vi "运维调试_总磷总氮.vi"() -> ()   [LabVIEW 2016, in "斯坦道总磷.lvlib"]
uses:
  <vilib>/Utility/miscctls.llb/LVStringsAndValuesArrayTypeDef_U16.ctl
  <vilib>/Utility/miscctls.llb/LVPointTypeDef.ctl
  <vilib>/Plasmionique/MB Master/MB_Master/MB_Master.lvclass
  <vilib>/Utility/config.llb/NI_LVConfig.lvlib
  <vilib>/ptbypt/NI_PtbyPt.lvlib
panel:
  in  "灯值调整":bool
  in  "测试量程配置":T1
  in  "启动参数设置":bool
  out "固件版本号":string
  in  "定时设置":cluster{"启动":bool, "控制命令":T2, "测量参数":T3}(xcontrol)
  out "模块版本号":string
  out "温度2":sgl
  out "温度1":sgl
  out "ADC":sgl
  out "F3":sgl format="%#.6f"
  out "F2":sgl format="%#.6f"
  out "F1":sgl format="%#.6f"
  out "F0":sgl format="%#.6f"
  out "运行状态":T4 {"数据时间:" format="%<%y/%m/%d %H:%M:%S>T"; "仪器时间:" format="%<%y/%m/%d %H:%M:%S>T"}
  in  "单选按钮":enum32{"COD", "NH3N", "TN", "TP"}(radio)=enum."TN"
  in  "仪器参数":bool
  out "二级权限":bool
  out "一级权限":bool
  out "输入密码":u32
  out "布尔":bool
  in  "流程固件":bool
  in  "量程参数读取":T5
  in  "模块启用":bool
  in  "串口设置":bool
  in  "公式一键写入":bool
  in  "流程路径":path=path "data/流程.xml"
  in  "曲线模型":cluster{"X^2":dbl, "X":dbl, "B":dbl, "r^2":dbl}(xcontrol)
  out "字符串 2":string
  in  "质控参数设置":bool
  in  "数组":string[](array[string])
  in  "量程切换阈值写入":bool
  in  "量程切换阈值读取":bool
  in  "参数下拉列表":enum16{"COD", "氨氮", "总氮", "总磷"}(ring)
  in  "量程下拉列表":enum16{"低量程", "高量程"}(ring)
  in  "测量模式下拉列表":enum16{"水样测量", "零点核查", "跨度核查", "标样核查", "加标回收"}(ring)
  in  "公式":cluster{"X^2":dbl, "X":dbl, "b":dbl}
  in  "写公式":bool
  in  "读公式":bool
  in  "返回":bool
  in  "参数设置":bool
  out "集成报警信息":string
  in  "停止":bool
  in  "手动启动":bool
  in  "单步测试":bool
  out "多列列表框":i32(listbox)
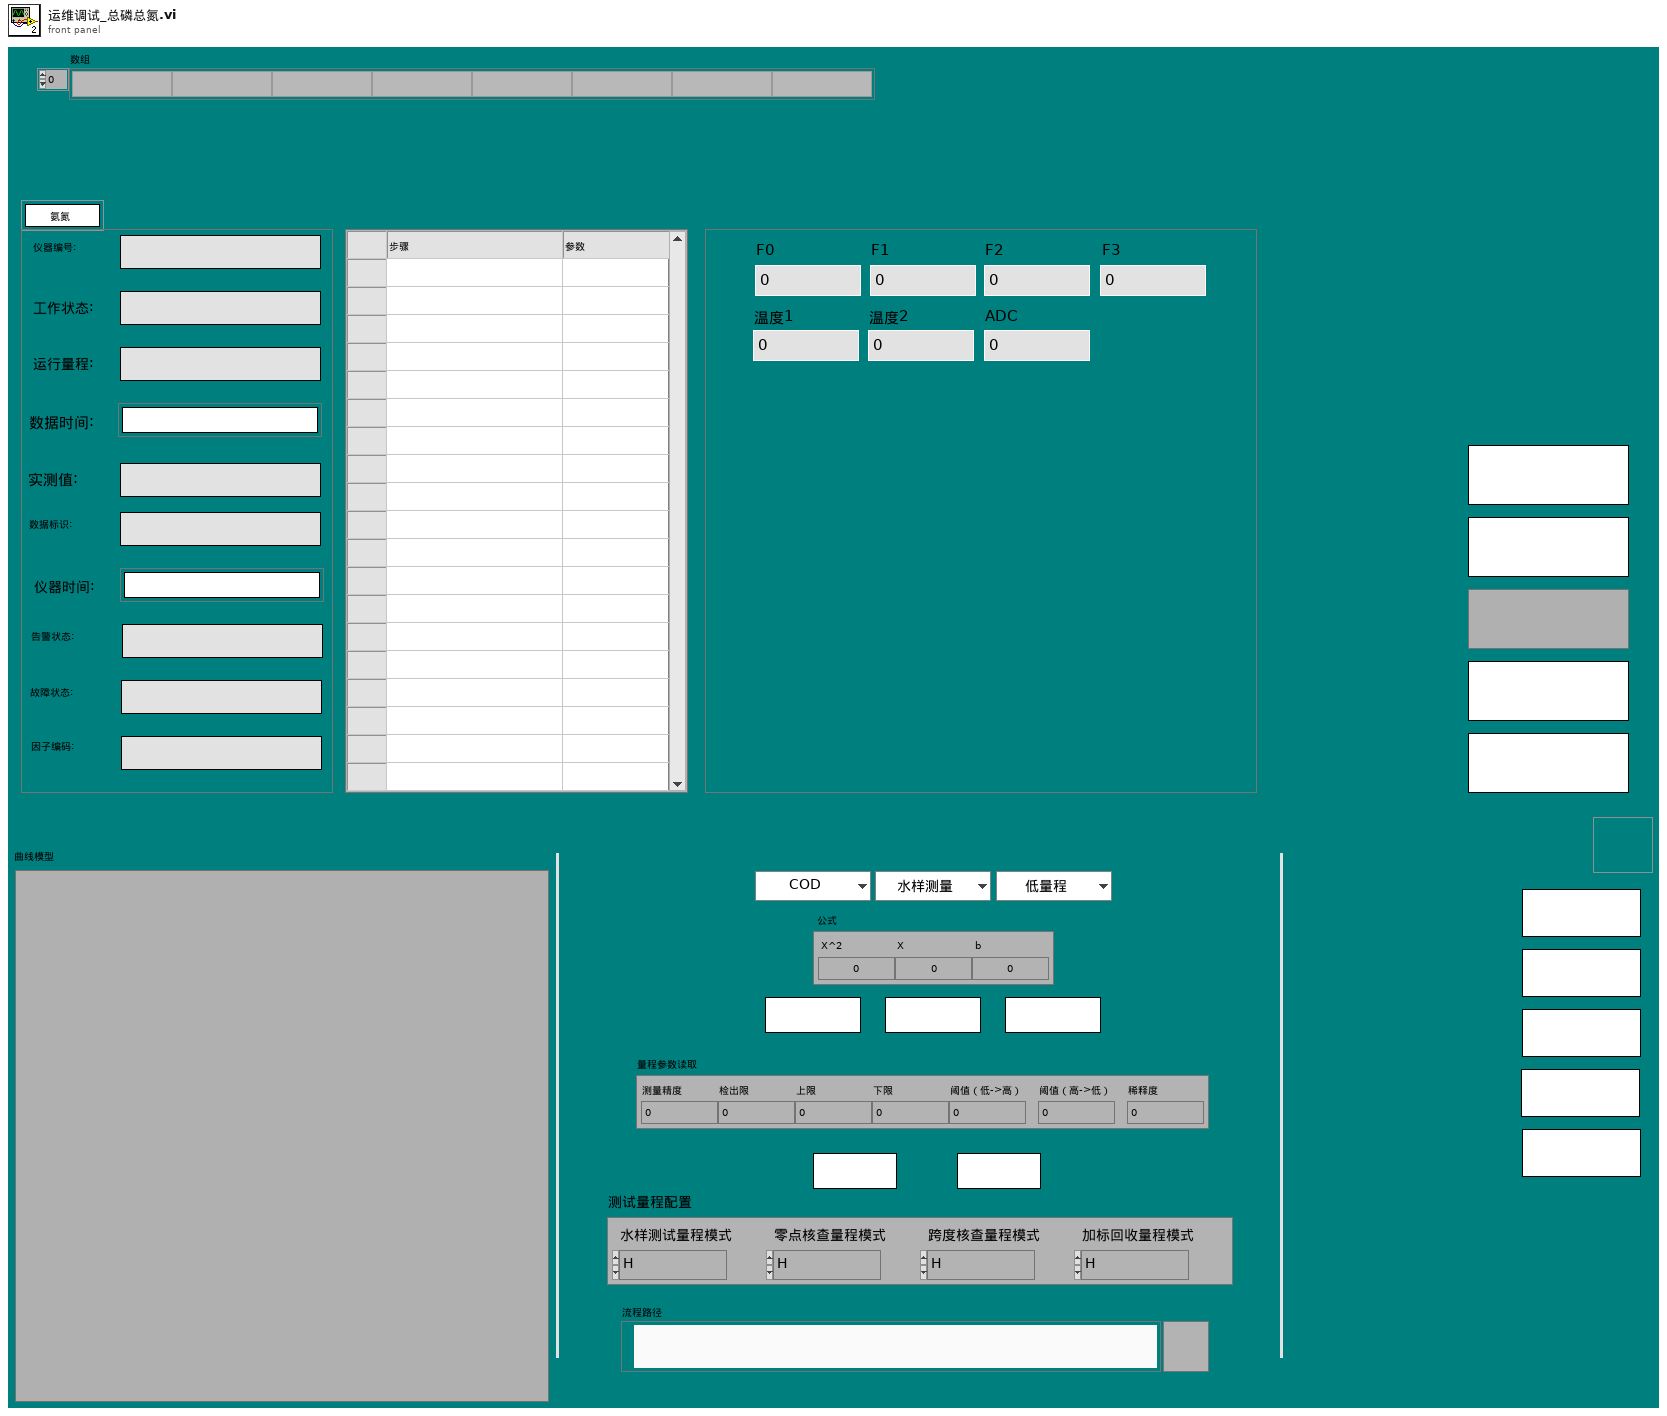
[diagram p1: front panel]
types:
  T1 = cluster{"水样测试量程模式":enum16{"H", "L", "AUTO"}, "空白核查量程模式":enum16{"H", "L", "AUTO"}, "跨度核查量程模式":enum16{"H", "L", "AUTO"}, "跨度核查量程模式 2":enum16{"H", "L", "AUTO"}}
  T2 = typedef "定时设置.xctl/国标控制命令.ctl" = enum16{"启动测量", "标样核查", "零点核查", "跨度核查", "空白测试", "平行样测试", "加标回收", "空白校准", "标样校准", "初始化（清洗）", "停止测试", "仪器重启", "校时", "模式设置", "测量间隔设置"}
  T3 = typedef "定时设置.xctl/测量参数.ctl" = u16
  T4 = cluster{"仪器编号:":string, "工作状态:":string, "运行量程: ":string, "数据时间:":timestamp, "实测值:":string, "数据标识: ":string, "仪器时间:":timestamp, "告警状态: ":string, "故障状态:  ":string, "因子编码:":string}
  T5 = cluster{"测量精度":dbl, "检出限":dbl, "上限":dbl, "下限":dbl, "阈值（低->高）":dbl, "阈值（高->低）":dbl, "稀释度":dbl}
  T6 = cluster{"时间源选择":enum16{"系统时间源", "仪器时间源"}, "外部时间源":timestamp}
  T7 = cluster{"系统时间":timestamp, "工作状态":enum16{"空闲", "水样测试", "标样核查", "零点核查", "跨度核查", "空白测试", "平行样测试", "加标回收", "空白校准", "标样校准", "初始化（清洗）"}, "测量模式":enum16{"待机", "连续模式", "周期模式", "定点模式", "受控模式", "手动模式"}, "告警代码":u16, "故障代码":u16, "日志代码":u16, "软件版本":u16, "F0":sgl, "F1":sgl, "F2":sgl, "F3":sgl, "T":sgl, "H":sgl, "id":u16, "flowid":u16, "量程":u16, "总磷控温温度1":sgl, "营养盐控温温度2":sgl, "ADC":sgl}
  T8 = enum32{"Bad", "Idle", "Run top level", "Running"}
  T9 = enum16{"空闲", "水样测试", "标样核查", "零点核查", "跨度核查", "空白测试", "平行样测试", "加标回收", "空白校准", "标样校准", "初始化（清洗）"}
  T10 = cluster{"水样测试量程模式":enum16{"H", "L", "AUTO"}, "空白核查量程模式":enum16{"H", "L", "AUTO"}, "跨度核查量程模式":enum16{"H", "L", "AUTO"}, "加标回收量程模式":enum16{"H", "L", "AUTO"}}
  T11 = typedef "LVStringsAndValuesArrayTypeDef_U16.ctl" = cluster{"String":string, "Value":u16}[]
  T12 = cluster{"COD":bool, "氨氮":bool, "总氮":bool, "总磷":bool}
  T13 = typedef "LVPointTypeDef.ctl" = cluster{"Horizontal":i16, "Vertical":i16}
  T14 = cluster{"因子编码":u32, "单位":u16, "标样参考值":sgl, "水样数据时间":timestamp, "水样实测值":sgl, "水样数据标识":string, "标样数据时间":timestamp, "标样实测值":sgl, "标样数据标识":string, "空白数据时间":timestamp, "空白实测值":sgl, "空白数据标识":string, "零点核查数据时间":timestamp, "零点核查实测值":sgl, "零点核查数据标识":string, "跨度核查数据时间":timestamp, "跨度核查实测值":sgl, "跨度核查数据标识":string, "加标回收数据时间":timestamp, "加标回收实测值":sgl, "加标回收数据标识":string, "平行样数据时间":timestamp, "平行样实测值":sgl, "平行样数据标识":string, "F0":sgl, "F1":sgl, "F2":sgl, "F3":sgl, "F4":sgl, "F5":sgl, "F6":sgl, "F7":sgl, "温度":sgl, "湿度":sgl, "X值":sgl, "fidrange":u16}
  T15 = cluster{"时间标识":timestamp, "设备":string, "日志信息":string, "备注":string}
  T16 = cluster{"参数":string, "报警内容":string, "报警分析":string}
  T17 = typedef "NI_LVConfig.lvlib/Config Data RefNum.ctl" = refnum<k1>
  T18 = cluster{"启动模式":enum16{"跨度核查", "水样测量", "空白核查", "标样核查", "加标回收"}, "启动参数":u16, "量程":enum16{"低量程", "高量程"}}
  T19 = cluster{"时间标识":timestamp, "设备":string, "日志信息":string, "流程参数":string}
  T20 = typedef "LVRowAndColumnUnsignedTypeDef.ctl" = cluster{"Row":u32, "Column":u32}
  T21 = cluster{"Major":u16, "Minor":u16, "Fix":u16, "Build":u16}
  T22 = cluster{"站号":u16, "量程切换":enum32{"H", "L", "AUTO"}, "控制命令":enum16{"启动测量", "标样核查", "零点核查", "跨度核查", "空白测试", "平行样测试", "加标回收", "空白校准", "标样校准", "初始化（清洗）", "停止测试", "仪器重启", "校时", "模式设置", "测量间隔设置"}, "模式设置":enum16{"待机", "连续模式", "周期模式", "定点模式", "受控模式", "手动模式"}, "测量间隔":u16}
  T23 = cluster{"参数下拉列表":enum16{"COD", "氨氮", "总氮", "总磷"}, "测量模式下拉列表":enum16{"水样测量", "零点核查", "跨度核查", "标样核查", "加标回收"}, "量程下拉列表":enum16{"低量程", "高量程"}}
  T24 = cluster{"被复制模型":cluster{"参数":u8, "测量模式":u8, "量程":u8}, "被覆盖模型":cluster{"参数":u8, "测量模式":u8, "量程":u8}[]}
  T25 = cluster{"总磷跨度值":dbl, "总磷零点标准液浓度":dbl, "总磷跨度标准液浓度":dbl, "总磷标准液标准浓度":dbl, "总氮跨度值":dbl, "总氮零点标准液浓度":dbl, "总氮跨度标准液浓度":dbl, "总氮标准液标准浓度":dbl, "COD跨度值":dbl, "COD零点标准液浓度":dbl, "COD跨度标准液浓度":dbl, "COD标准液标准浓度":dbl, "氨氮跨度值":dbl, "氨氮零点标准液浓度":dbl, "氨氮跨度标准液浓度":dbl, "氨氮标准液标准浓度":dbl}
  T26 = cluster{"测量量程":dbl, "测量精度":dbl, "测量间隔":dbl, "消解温度":dbl, "消解时长":dbl, "空白校准时间":timestamp, "曲线截距":dbl, "曲线斜率":dbl, "测量检出限":dbl, "测量信号值":dbl, "线性相关系数":dbl, "二次多项式系数":dbl, "标样校准时间":timestamp, "稀释倍数":dbl, "三项式系数":dbl, "空白标定系数":dbl, "量程系数":dbl, "F0/ORPA":dbl, "F1/ORPB":dbl, "F2/ORPK":dbl, "F3":dbl, "F4":dbl, "F5":dbl, "F6":dbl, "F7":dbl, "X0/滴定数":dbl, "量程":dbl}
  T27 = cluster{"COD仪器参数":cluster{"测量量程":dbl, "测量精度":dbl, "测量间隔":dbl, "消解温度":dbl, "消解时长":dbl, "空白校准时间":timestamp, "曲线截距":dbl, "曲线斜率":dbl, "测量检出限":dbl, "测量信号值":dbl, "线性相关系数":dbl, "二次多项式系数":dbl, "标样校准时间":timestamp, "稀释倍数":dbl, "三项式系数":dbl, "空白标定系数":dbl, "量程系数":dbl, "F0/ORPA":dbl, "F1/ORPB":dbl, "F2/ORPK":dbl, "F3":dbl, "F4":dbl, "F5":dbl, "F6":dbl, "F7":dbl, "X0/滴定数":dbl, "量程":dbl}, "氨氮仪器参数":cluster{"测量量程":dbl, "测量精度":dbl, "测量间隔":dbl, "消解温度":dbl, "消解时长":dbl, "空白校准时间":timestamp, "曲线截距":dbl, "曲线斜率":dbl, "测量检出限":dbl, "测量信号值":dbl, "线性相关系数":dbl, "二次多项式系数":dbl, "标样校准时间":timestamp, "稀释倍数":dbl, "三项式系数":dbl, "空白标定系数":dbl, "量程系数":dbl, "F0/ORPA":dbl, "F1/ORPB":dbl, "F2/ORPK":dbl, "F3":dbl, "F4":dbl, "F5":dbl, "F6":dbl, "F7":dbl, "X0/滴定数":dbl, "量程":dbl}, "总氮仪器参数":cluster{"测量量程":dbl, "测量精度":dbl, "测量间隔":dbl, "消解温度":dbl, "消解时长":dbl, "空白校准时间":timestamp, "曲线截距":dbl, "曲线斜率":dbl, "测量检出限":dbl, "测量信号值":dbl, "线性相关系数":dbl, "二次多项式系数":dbl, "标样校准时间":timestamp, "稀释倍数":dbl, "三项式系数":dbl, "空白标定系数":dbl, "量程系数":dbl, "F0/ORPA":dbl, "F1/ORPB":dbl, "F2/ORPK":dbl, "F3":dbl, "F4":dbl, "F5":dbl, "F6":dbl, "F7":dbl, "X0/滴定数":dbl, "量程":dbl}, "总磷仪器参数":cluster{"测量量程":dbl, "测量精度":dbl, "测量间隔":dbl, "消解温度":dbl, "消解时长":dbl, "空白校准时间":timestamp, "曲线截距":dbl, "曲线斜率":dbl, "测量检出限":dbl, "测量信号值":dbl, "线性相关系数":dbl, "二次多项式系数":dbl, "标样校准时间":timestamp, "稀释倍数":dbl, "三项式系数":dbl, "空白标定系数":dbl, "量程系数":dbl, "F0/ORPA":dbl, "F1/ORPB":dbl, "F2/ORPK":dbl, "F3":dbl, "F4":dbl, "F5":dbl, "F6":dbl, "F7":dbl, "X0/滴定数":dbl, "量程":dbl}}
  T28 = cluster{"测量精度":u16, "检出限":dbl, "上限":dbl, "下限":dbl, "阈值（低->高）":dbl, "阈值（高->低）":dbl, "稀释度":dbl}
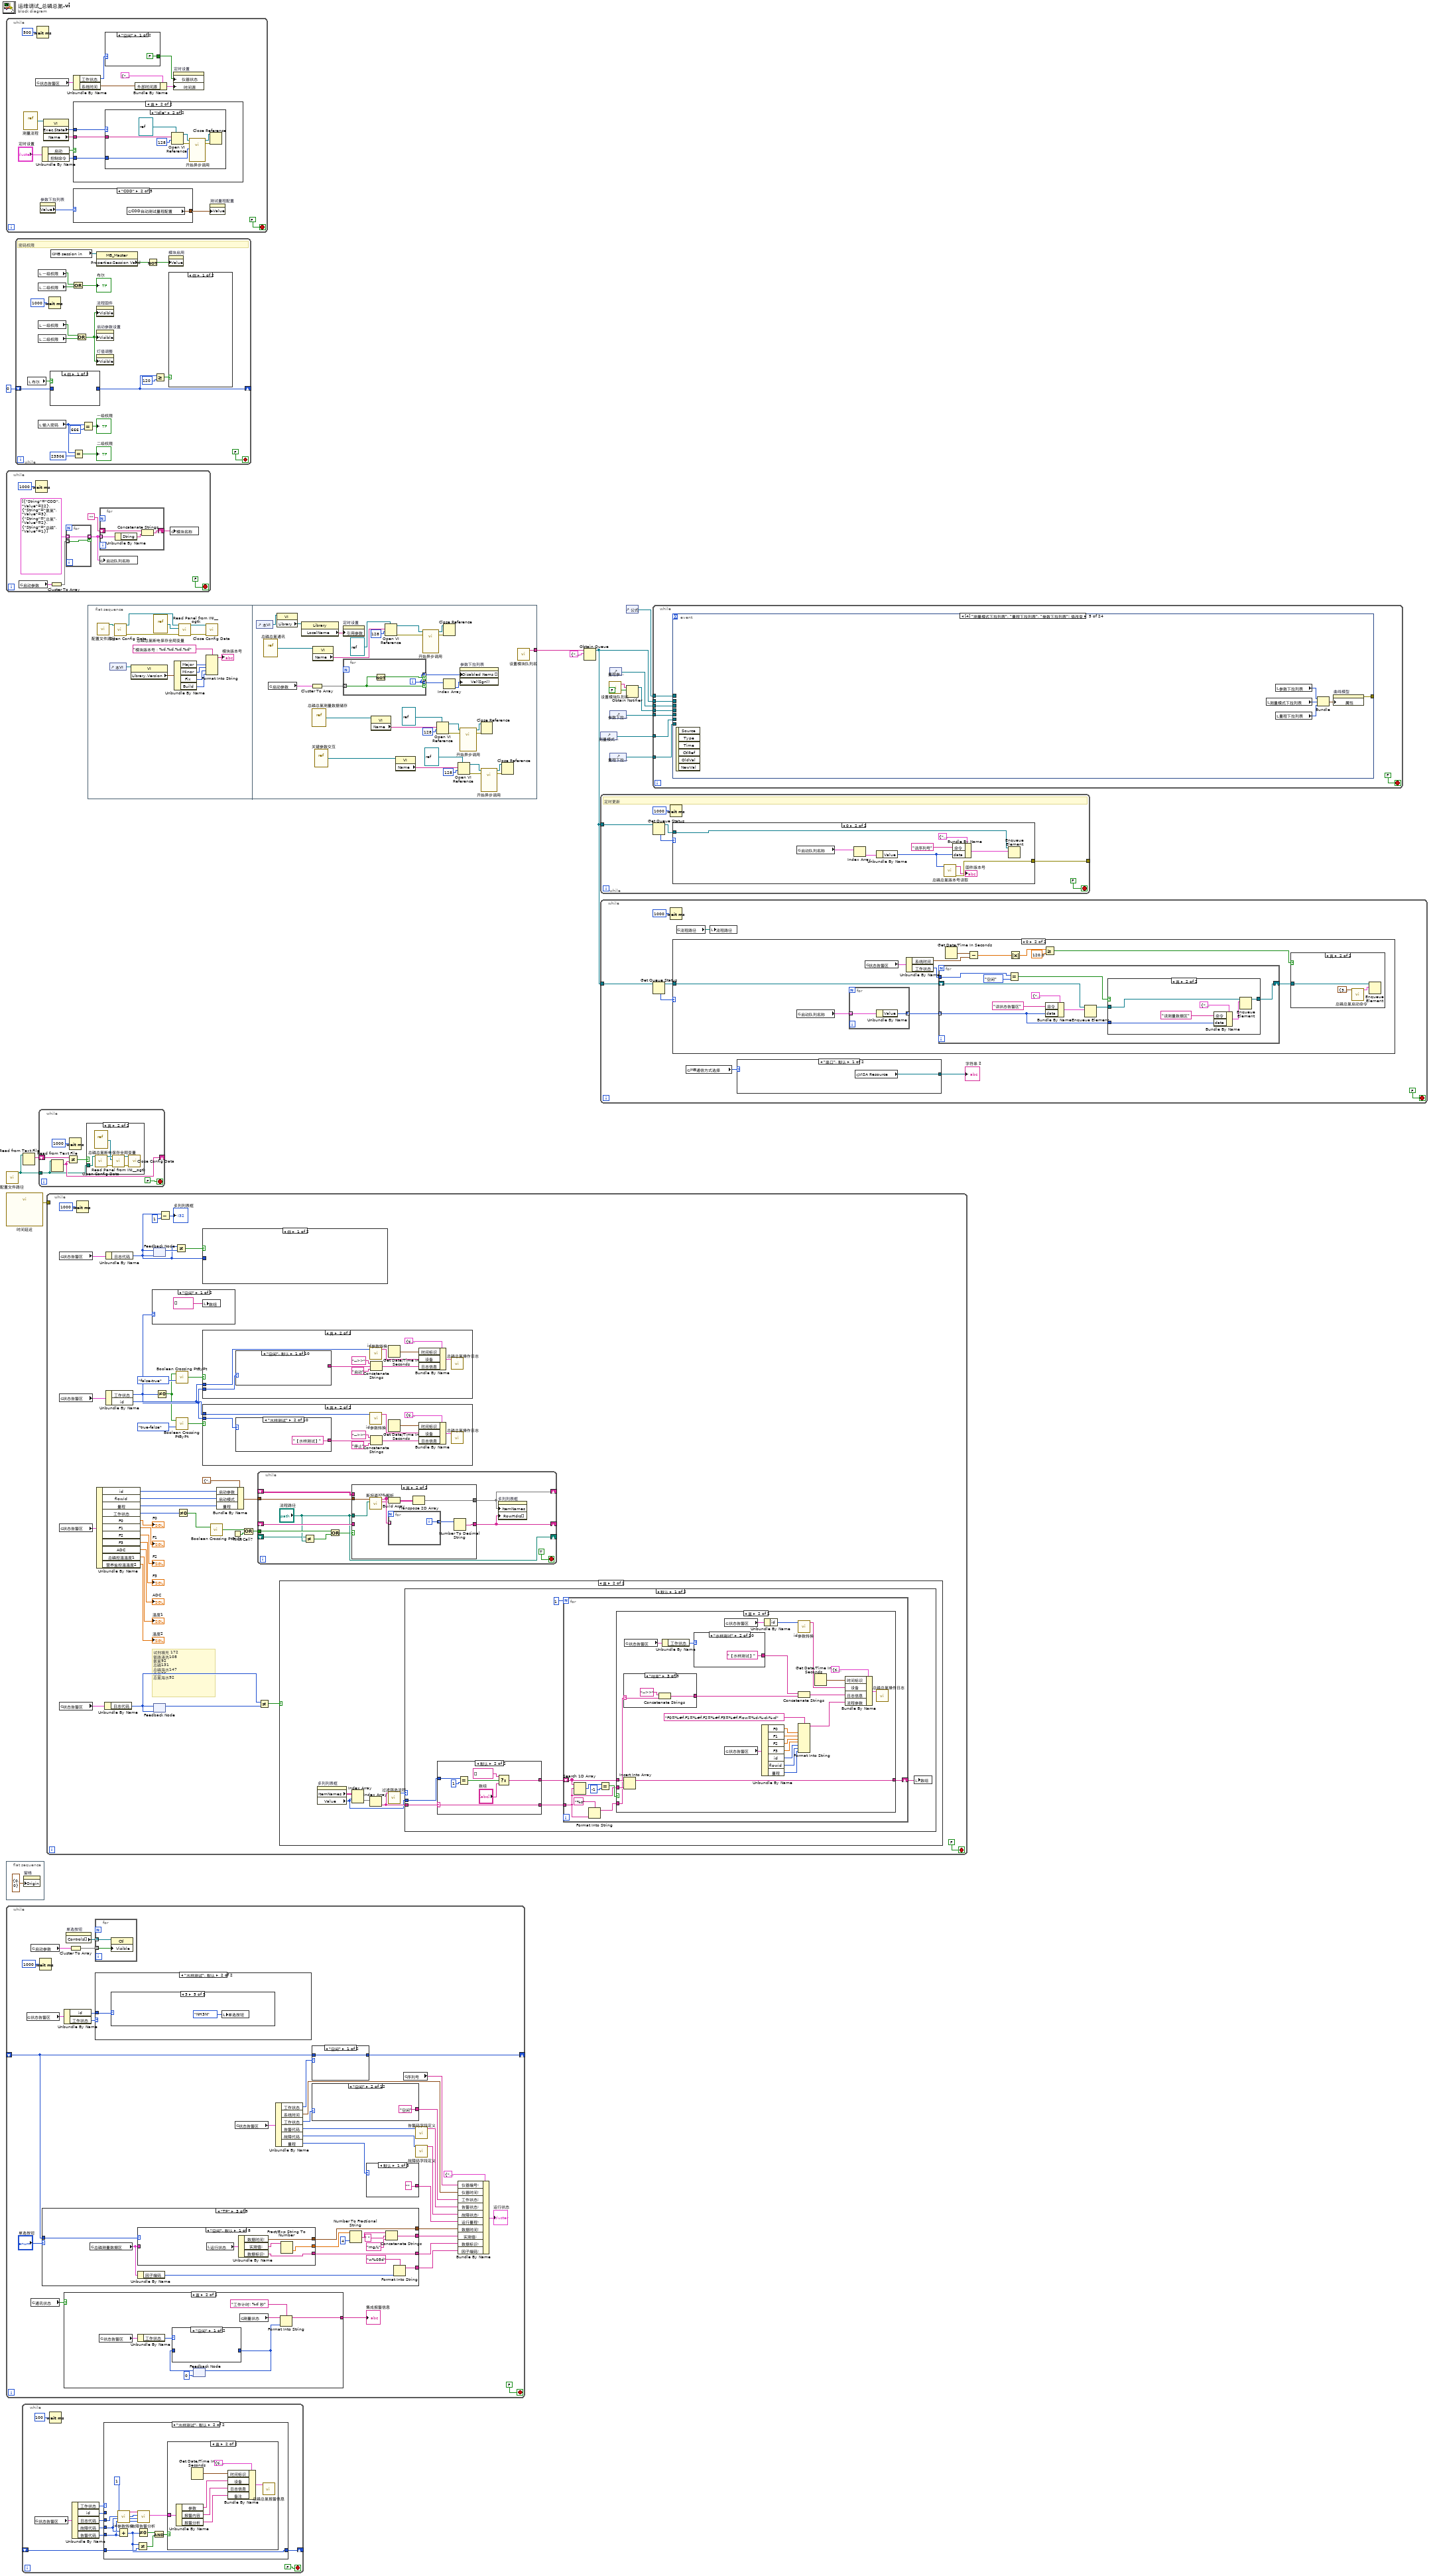
[diagram p0: block diagram]
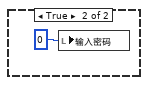
[diagram p5: hidden frame]
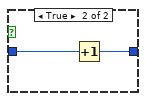
[diagram p6: hidden frame]
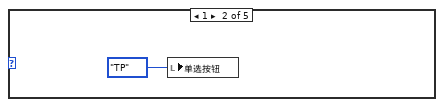
[diagram p11: hidden frame]
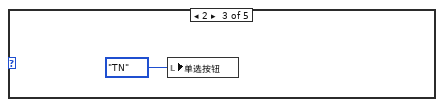
[diagram p12: hidden frame]
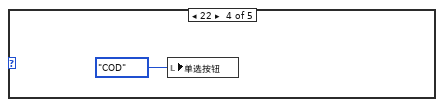
[diagram p13: hidden frame]
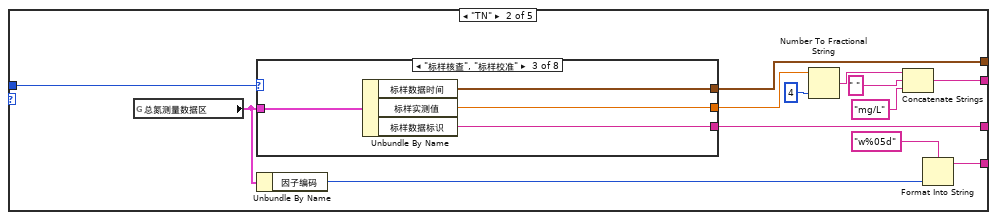
[diagram p15: hidden frame]
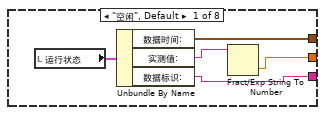
[diagram p16: hidden frame]
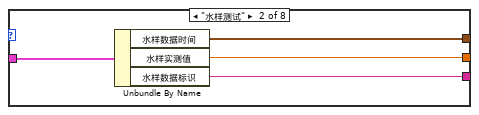
[diagram p17: hidden frame]
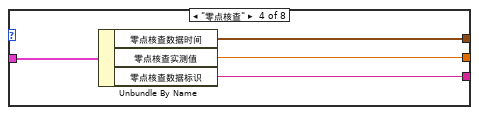
[diagram p18: hidden frame]
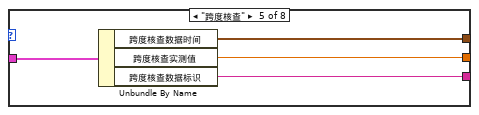
[diagram p19: hidden frame]
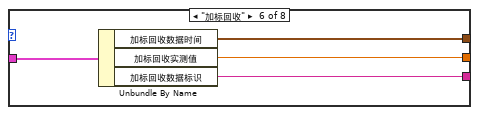
[diagram p20: hidden frame]
diagram:
  n1 = while {
    stop <- FALSE stop-if-true
    n2 = vi-ref "测量流程.vi"() -> (w29:refnum<vi>)
    n3 = global read "VAR总磷总氮全局变量.vi" "状态告警区"() -> (w26:T7)
    n4 = Wait (ms)(milliseconds to wait=u32 500 ("等待时间（毫秒）")) -> ()  [unwired: 1 out]
    n5 = property on="参数下拉列表" class="Enum (严格)"() -> ("Value"=w18:enum16{"COD", "氨氮", "总氮", "总磷"})  [unwired: 2 in, 2 out]
    n6 = Unbundle By Name("定时设置") -> ("启动"=w23:bool, "控制命令"=w22:T2)
    n7 = property class="VI"(reference=w29) -> ("Exec.State"=w28:T8, "Name"=w27:string)  [unwired: 1 in, 2 out]
    n8 = Unbundle By Name(w26) -> ("工作状态"=w25:T9, "系统时间"=w20:timestamp)
    n9 = case shown="真" w23 {
      tunnel: w27 -> [_ w40]
      tunnel: w22 -> [_ w39]
      tunnel: w28 -> [_ w38]
      frame False {
      }
      frame True {
        n10 = case shown="\"Idle\"" w38 {
          tunnel: w40 -> [_ w44]
          tunnel: w39 -> [_ w41]
          frame "Bad", Default {
          }
          frame "Idle" {
            n11 = Open VI Reference(type specifier VI Refnum (for type only)=refnum<vi> refnum, vi path=w44, options=128 ("选项")) -> (vi reference=w45:refnum<vi>, error out=w46:errorcluster)  [unwired: 3 in]
            n12 = call-by-ref "开始异步调用"(reference=w45, error in=w46, "控制命令"=w41) -> (reference out=w47:refnum<vi>, error out=w48:errorcluster)  [unwired: 11 in]
            n13 = Close Reference(reference=w47, error in (no error)=w48) -> ()  [unwired: 1 out]
          }
        }
      }
    }
    n14 = case shown="\"COD\"" w18 {
      tunnel: [_ w32 w33 w34 w35] -> w17
      frame Default {
      }
      frame "COD" {
        n15 = global read "总磷总氮断电保存全局变量.vi" "COD自动测试量程配置"() -> (w32:T10)
      }
      frame "氨氮" {
        n16 = global read "总磷总氮断电保存全局变量.vi" "氨氮自动测试量程配置"() -> (w33:T10)
      }
      frame "总氮" {
        n17 = global read "总磷总氮断电保存全局变量.vi" "总氮自动测试量程配置"() -> (w34:T10)
      }
      frame "总磷" {
        n18 = global read "总磷总氮断电保存全局变量.vi" "总磷自动测试量程配置"() -> (w35:T10)
      }
    }
    n19 = case shown="\"空闲\"" w25 {
      tunnel: [FALSE TRUE] -> w16
      frame "空闲" {
      }
      frame "水样测试", Default {
      }
    }
    n20 = Bundle By Name(cluster=T6 {"时间源选择"=enum."仪器时间源", "外部时间源"=timestamp(0 s since 1904-01-01)} ("时间源"), "外部时间源"=w20) -> (w19:T6)
    n21 = property on="定时设置" class="定时设置 (严格)"("仪器状态"=w16, "时间源"=w19) -> ()  [unwired: 2 in, 2 out]
    n22 = property on="测试量程配置" class="Clust (严格)"("Value"=w17) -> ()  [unwired: 2 in, 2 out]
  }
  n23 = while {
    stop <- FALSE stop-if-true
    n24 = global read "总磷总氮断电保存全局变量.vi" "启动参数"() -> (w54:T12)
    n25 = Wait (ms)(milliseconds to wait=u32 1000 ("等待时间（毫秒）")) -> ()  [unwired: 1 out]
    n26 = Cluster To Array(cluster=w54) -> (array=w53:bool[])
    n27 = for {
      tunnel: w53 -> [w62] mode=indexing
      tunnel: T11 [{"String"="COD", "Value"=22}, {"String"="氨氮", "Value"=3}, {"String"="总氮", "Value"=2}, {"String"="总磷", "Value"=1}] ("字符串与值[]") -> [w61] mode=indexing
      tunnel: [w61] -> w51 mode=indexing if=w62
    }
    n28 = for {
      tunnel: w51 -> [w60] mode=indexing
      shift-right: [w59] -> w49
      shift-left: "" -> [w57]
      n29 = Unbundle By Name(w60) -> ("String"=w58:string)
      n30 = Concatenate Strings(w57, w58) -> (w59:string)
    }
    n31 = global write "VAR总磷总氮全局变量.vi" "启动队列名称"(w51) -> ()
    n32 = global write "VAR总磷总氮全局变量.vi" "模块名称"(w49) -> ()
  }
  n33 = call "配置文件路径.vi"() -> ("appended path"=w4:path)  [unwired: 11 in]
  n34 = call "时间延迟"() -> ("error out"=w10:errorcluster)  [unwired: 11 in]
  n35 = flat-sequence {
    frame #0 {
      n36 = property on="窗格" class="Pane"("Origin"=T13 {"Horizontal"=0, "Vertical"=0} ("原点")) -> ()  [unwired: 2 in, 2 out]
    }
  }
  n37 = while {
    shift-right: [w65] -> _
    shift-left: _ -> [w64]
    stop <- FALSE stop-if-true
    n38 = global read "VAR总磷总氮全局变量.vi" "状态告警区"() -> (w76:T7)
    n39 = global read "总磷总氮断电保存全局变量.vi" "启动参数"() -> (w68:T12)
    n40 = global read "VAR总磷总氮全局变量.vi" "通讯状态"() -> (w92:bool)
    n41 = Wait (ms)(milliseconds to wait=u32 1000 ("等待时间（毫秒）")) -> ()  [unwired: 1 out]
    n42 = case shown="\"TP\"" "单选按钮" {
      tunnel: w64 -> [_ w108 w154 w200 w246]
      tunnel: [_ w107 w153 w198 w244] -> w80
      tunnel: [_ w106 w156 w202 w248] -> w79
      tunnel: [_ w105 w151 w196 w242] -> w78
      tunnel: [_ w104 w155 w201 w247] -> w77
      frame Default {
      }
      frame "TN" {
        n43 = global read "VAR总磷总氮全局变量.vi" "总氮测量数据区"() -> (w109:T14)
        n44 = case shown="\"标样核查\", \"标样校准\"" w108 {
          tunnel: [w119 w125 w129 w133 w137 w141 w145 w149] -> w107
          tunnel: [w117 w124 w128 w132 w135 w140 w144 w148] -> w111
          tunnel: [w120 w123 w127 w131 w134 w139 w143 w147] -> w105
          tunnel: w109 -> [_ w122 w126 w130 w136 w138 w142 w146]
          frame "空闲", Default {
            n45 = local read "运行状态"() -> (w121:T4)
            n46 = Unbundle By Name(w121) -> ("数据时间:"=w119:timestamp, "实测值:"=w118:string, "数据标识:"=w120:string)
            n47 = Fract/Exp String To Number(string=w118) -> (number=w117:dbl)  [unwired: 3 in, 1 out]
          }
          frame "水样测试" {
            n48 = Unbundle By Name(w122) -> ("水样数据时间"=w125:timestamp, "水样实测值"=w124:sgl, "水样数据标识"=w123:string)
          }
          frame "标样核查", "标样校准" {
            n49 = Unbundle By Name(w126) -> ("标样数据时间"=w129:timestamp, "标样实测值"=w128:sgl, "标样数据标识"=w127:string)
          }
          frame "零点核查" {
            n50 = Unbundle By Name(w130) -> ("零点核查数据时间"=w133:timestamp, "零点核查实测值"=w132:sgl, "零点核查数据标识"=w131:string)
          }
          frame "跨度核查" {
            n51 = Unbundle By Name(w136) -> ("跨度核查数据时间"=w137:timestamp, "跨度核查实测值"=w135:sgl, "跨度核查数据标识"=w134:string)
          }
          frame "加标回收" {
            n52 = Unbundle By Name(w138) -> ("加标回收数据时间"=w141:timestamp, "加标回收实测值"=w140:sgl, "加标回收数据标识"=w139:string)
          }
          frame "空白测试", "空白校准" {
            n53 = Unbundle By Name(w142) -> ("空白数据时间"=w145:timestamp, "空白实测值"=w144:sgl, "空白数据标识"=w143:string)
          }
          frame "平行样测试" {
            n54 = Unbundle By Name(w146) -> ("平行样数据时间"=w149:timestamp, "平行样实测值"=w148:sgl, "平行样数据标识"=w147:string)
          }
        }
        n55 = Unbundle By Name(w109) -> ("因子编码"=w115:u32)
        n56 = Number To Fractional String(number=w111, precision (6)=i16 4 ("精度(6)")) -> (F-format string=w113:string)  [unwired: 2 in]
        n57 = Concatenate Strings(w113, " " ("字符串"), "mg/L" ("字符串")) -> (w106:string)
        n58 = Format Into String(format string="w%05d" ("格式字符串"), w115) -> (resulting string=w104:string)  [unwired: 2 in, 1 out]
      }
      frame "TP" {
        n59 = global read "VAR总磷总氮全局变量.vi" "总磷测量数据区"() -> (w150:T14)
        n60 = case shown="\"空闲\", 默认" w154 {
          tunnel: [w165 w171 w175 w179 w183 w187 w191 w195] -> w153
          tunnel: [w163 w170 w174 w178 w181 w186 w190 w194] -> w152
          tunnel: [w166 w169 w173 w177 w180 w185 w189 w193] -> w151
          tunnel: w150 -> [_ w168 w172 w176 w182 w184 w188 w192]
          frame "空闲", Default {
            n61 = local read "运行状态"() -> (w167:T4)
            n62 = Unbundle By Name(w167) -> ("数据时间:"=w165:timestamp, "实测值:"=w164:string, "数据标识:"=w166:string)
            n63 = Fract/Exp String To Number(string=w164) -> (number=w163:dbl)  [unwired: 3 in, 1 out]
          }
          frame "水样测试" {
            n64 = Unbundle By Name(w168) -> ("水样数据时间"=w171:timestamp, "水样实测值"=w170:sgl, "水样数据标识"=w169:string)
          }
          frame "标样核查" {
            n65 = Unbundle By Name(w172) -> ("标样数据时间"=w175:timestamp, "标样实测值"=w174:sgl, "标样数据标识"=w173:string)
          }
          frame "零点核查" {
            n66 = Unbundle By Name(w176) -> ("零点核查数据时间"=w179:timestamp, "零点核查实测值"=w178:sgl, "零点核查数据标识"=w177:string)
          }
          frame "跨度核查" {
            n67 = Unbundle By Name(w182) -> ("跨度核查数据时间"=w183:timestamp, "跨度核查实测值"=w181:sgl, "跨度核查数据标识"=w180:string)
          }
          frame "加标回收" {
            n68 = Unbundle By Name(w184) -> ("加标回收数据时间"=w187:timestamp, "加标回收实测值"=w186:sgl, "加标回收数据标识"=w185:string)
          }
          frame "空白测试" {
            n69 = Unbundle By Name(w188) -> ("空白数据时间"=w191:timestamp, "空白实测值"=w190:sgl, "空白数据标识"=w189:string)
          }
          frame "平行样测试" {
            n70 = Unbundle By Name(w192) -> ("平行样数据时间"=w195:timestamp, "平行样实测值"=w194:sgl, "平行样数据标识"=w193:string)
          }
        }
        n71 = Unbundle By Name(w150) -> ("因子编码"=w161:u32)
        n72 = Number To Fractional String(number=w152, precision (6)=i16 4 ("精度(6)")) -> (F-format string=w159:string)  [unwired: 2 in]
        n73 = Concatenate Strings(w159, " " ("字符串"), "mg/L" ("字符串")) -> (w156:string)
        n74 = Format Into String(format string="w%05d" ("格式字符串"), w161) -> (resulting string=w155:string)  [unwired: 2 in, 1 out]
      }
      frame "NH3N" {
        n75 = global read "VAR总磷总氮全局变量.vi" "氨氮测量数据区"() -> (w199:T14)
        n76 = case shown="\"空闲\", 默认" w200 {
          tunnel: [w211 w217 w221 w225 w229 w233 w237 w241] -> w198
          tunnel: [w209 w216 w220 w224 w227 w232 w236 w240] -> w197
          tunnel: [w212 w215 w219 w223 w226 w231 w235 w239] -> w196
          tunnel: w199 -> [_ w214 w218 w222 w228 w230 w234 w238]
          frame "空闲", Default {
            n77 = local read "运行状态"() -> (w213:T4)
            n78 = Unbundle By Name(w213) -> ("数据时间:"=w211:timestamp, "实测值:"=w210:string, "数据标识:"=w212:string)
            n79 = Fract/Exp String To Number(string=w210) -> (number=w209:dbl)  [unwired: 3 in, 1 out]
          }
          frame "水样测试" {
            n80 = Unbundle By Name(w214) -> ("水样数据时间"=w217:timestamp, "水样实测值"=w216:sgl, "水样数据标识"=w215:string)
          }
          frame "标样核查" {
            n81 = Unbundle By Name(w218) -> ("标样数据时间"=w221:timestamp, "标样实测值"=w220:sgl, "标样数据标识"=w219:string)
          }
          frame "零点核查" {
            n82 = Unbundle By Name(w222) -> ("零点核查数据时间"=w225:timestamp, "零点核查实测值"=w224:sgl, "零点核查数据标识"=w223:string)
          }
          frame "跨度核查" {
            n83 = Unbundle By Name(w228) -> ("跨度核查数据时间"=w229:timestamp, "跨度核查实测值"=w227:sgl, "跨度核查数据标识"=w226:string)
          }
          frame "加标回收" {
            n84 = Unbundle By Name(w230) -> ("加标回收数据时间"=w233:timestamp, "加标回收实测值"=w232:sgl, "加标回收数据标识"=w231:string)
          }
          frame "空白测试" {
            n85 = Unbundle By Name(w234) -> ("空白数据时间"=w237:timestamp, "空白实测值"=w236:sgl, "空白数据标识"=w235:string)
          }
          frame "平行样测试" {
            n86 = Unbundle By Name(w238) -> ("平行样数据时间"=w241:timestamp, "平行样实测值"=w240:sgl, "平行样数据标识"=w239:string)
          }
        }
        n87 = Unbundle By Name(w199) -> ("因子编码"=w207:u32)
        n88 = Number To Fractional String(number=w197, precision (6)=i16 4 ("精度(6)")) -> (F-format string=w205:string)  [unwired: 2 in]
        n89 = Concatenate Strings(w205, " " ("字符串"), "mg/L" ("字符串")) -> (w202:string)
        n90 = Format Into String(format string="w%05d" ("格式字符串"), w207) -> (resulting string=w201:string)  [unwired: 2 in, 1 out]
      }
      frame "COD" {
        n91 = global read "VAR总磷总氮全局变量.vi" "COD测量数据区"() -> (w245:T14)
        n92 = case shown="\"空闲\", 默认" w246 {
          tunnel: [w257 w263 w267 w271 w275 w279 w283 w287] -> w244
          tunnel: [w255 w262 w266 w270 w273 w278 w282 w286] -> w243
          tunnel: [w258 w261 w265 w269 w272 w277 w281 w285] -> w242
          tunnel: w245 -> [_ w260 w264 w268 w274 w276 w280 w284]
          frame "空闲", Default {
            n93 = local read "运行状态"() -> (w259:T4)
            n94 = Unbundle By Name(w259) -> ("数据时间:"=w257:timestamp, "实测值:"=w256:string, "数据标识:"=w258:string)
            n95 = Fract/Exp String To Number(string=w256) -> (number=w255:dbl)  [unwired: 3 in, 1 out]
          }
          frame "水样测试" {
            n96 = Unbundle By Name(w260) -> ("水样数据时间"=w263:timestamp, "水样实测值"=w262:sgl, "水样数据标识"=w261:string)
          }
          frame "标样核查" {
            n97 = Unbundle By Name(w264) -> ("标样数据时间"=w267:timestamp, "标样实测值"=w266:sgl, "标样数据标识"=w265:string)
          }
          frame "零点核查" {
            n98 = Unbundle By Name(w268) -> ("零点核查数据时间"=w271:timestamp, "零点核查实测值"=w270:sgl, "零点核查数据标识"=w269:string)
          }
          frame "跨度核查" {
            n99 = Unbundle By Name(w274) -> ("跨度核查数据时间"=w275:timestamp, "跨度核查实测值"=w273:sgl, "跨度核查数据标识"=w272:string)
          }
          frame "加标回收" {
            n100 = Unbundle By Name(w276) -> ("加标回收数据时间"=w279:timestamp, "加标回收实测值"=w278:sgl, "加标回收数据标识"=w277:string)
          }
          frame "空白测试" {
            n101 = Unbundle By Name(w280) -> ("空白数据时间"=w283:timestamp, "空白实测值"=w282:sgl, "空白数据标识"=w281:string)
          }
          frame "平行样测试" {
            n102 = Unbundle By Name(w284) -> ("平行样数据时间"=w287:timestamp, "平行样实测值"=w286:sgl, "平行样数据标识"=w285:string)
          }
        }
        n103 = Unbundle By Name(w245) -> ("因子编码"=w253:u32)
        n104 = Number To Fractional String(number=w243, precision (6)=i16 4 ("精度(6)")) -> (F-format string=w251:string)  [unwired: 2 in]
        n105 = Concatenate Strings(w251, " " ("字符串"), "mg/L" ("字符串")) -> (w248:string)
        n106 = Format Into String(format string="w%05d" ("格式字符串"), w253) -> (resulting string=w247:string)  [unwired: 2 in, 1 out]
      }
    }
    n107 = Unbundle By Name(w76) -> ("id"=w75:u16, "工作状态"=w70:T9)
    n108 = case shown="真" w92 {
      tunnel: ["通讯异常" ("集成报警信息") w308] -> w91
      frame False {
      }
      frame True {
        n109 = global read "VAR总磷总氮全局变量.vi" "状态告警区"() -> (w314:T7)
        n110 = Unbundle By Name(w314) -> ("工作状态"=w313:T9)
        n111 = feedback #1(0) -> (w311:i32)
        n112 = case shown="\"空闲\"" w313 {
          tunnel: w311 -> [_ w316]
          tunnel: [_ w315] -> w309
          frame "空闲" {
          }
          frame Default {
            n113 = Increment(x=w316) -> (x+1=w315:i32)
          }
        }
        n114 = feedback-in #1(w309) -> ()
        n115 = global read "VAR总磷总氮全局变量.vi" "测量状态"() -> (w307:string)
        n116 = Format Into String(format string="工作计时: %d 秒" ("格式字符串"), initial string=w307, w309) -> (resulting string=w308:string)  [unwired: 1 in, 1 out]
      }
    }
    "集成报警信息" <- w91
    n117 = property on="单选按钮" class="RadioBtnsControl (严格)"() -> ("Controls[]"=w69:refnum<vi>[])  [unwired: 2 in, 2 out]
    n118 = Cluster To Array(cluster=w68) -> (array=w67:bool[])
    n119 = for {
      tunnel: w69 -> [w98] mode=indexing
      tunnel: w67 -> [w97] mode=indexing
      n120 = property class="Ctl"(reference=w98, "Visible"=w97) -> ()  [unwired: 1 in, 2 out]
    }
    n121 = case shown="\"水样测试\", 默认" w70 {
      tunnel: w75 -> [_ w99]
      frame "空闲" {
      }
      frame "水样测试", Default {
        n122 = case shown="3" w99 {
          frame 0, Default {
          }
          frame 1 {
            n123 = local write "单选按钮"(enum32{"COD", "NH3N", "TN", "TP"}."TP" ("单选按钮")) -> ()
          }
          frame 2 {
            n124 = local write "单选按钮"(enum32{"COD", "NH3N", "TN", "TP"}."TN" ("单选按钮")) -> ()
          }
          frame 22 {
            n125 = local write "单选按钮"(enum32{"COD", "NH3N", "TN", "TP"}."COD" ("单选按钮")) -> ()
          }
          frame 3 {
            n126 = local write "单选按钮"(enum32{"COD", "NH3N", "TN", "TP"}."NH3N" ("单选按钮")) -> ()
          }
        }
      }
    }
    n127 = global read "VAR总磷总氮全局变量.vi" "状态告警区"() -> (w90:T7)
    n128 = Unbundle By Name(w90) -> ("工作状态"=w66:T9, "系统时间"=w86:timestamp, "工作状态"=w85:T9, "告警代码"=w74:u16, "故障代码"=w72:u16, "量程"=w83:u16)
    n129 = case shown="\"空闲\"" w66 {
      selector: w66 -> [_ w96]
      tunnel: [w95 w96] -> w65
      tunnel: w64 -> [w95 _]
      frame "空闲" {
      }
      frame "水样测试", Default {
      }
    }
    n130 = case shown="\"空闲\"" w85 {
      selector: w85 -> [w291 _ _ _ _ _ _ _ _ _ _ _]
      tunnel: [w292 "空闲" ("工作状态") "水样测量" ("工作状态") "标样核查" ("工作状态") "零点核查" ("工作状态") "跨度核查" ("工作状态") "空白测试" ("工作状态") "平行样测试" ("工作状态") "加标回收" ("工作状态") "空白校准" ("工作状态") "标样校准" ("工作状态") "初始化" ("工作状态")] -> w84
      frame Default {
        n131 = Format Into String(format string="%d" ("格式字符串"), initial string="未知" ("工作状态"), w291) -> (resulting string=w292:string)  [unwired: 1 in, 1 out]
      }
      frame "空闲" {
      }
      frame "水样测试" {
      }
      frame "标样核查" {
      }
      frame "零点核查" {
      }
      frame "跨度核查" {
      }
      frame "空白测试" {
      }
      frame "平行样测试" {
      }
      frame "加标回收" {
      }
      frame "空白校准" {
      }
      frame "标样校准" {
      }
      frame "初始化（清洗）" {
      }
    }
    n132 = case shown="默认" w83 {
      tunnel: ["" ("字符串") "低量程" ("字符串") "高量程" ("字符串")] -> w82
      frame Default {
      }
      frame 0 {
      }
      frame 1 {
      }
    }
    n133 = global read "VAR总磷总氮全局变量.vi" "序列号"() -> (w87:string)
    n134 = call "告警码字段定义.vi"("告警代码"=w74) -> ("字符串"=w73:string)  [unwired: 8 in, 2 out]
    n135 = call "故障码字段定义.vi"("故障代码"=w72) -> ("字符串"=w71:string)  [unwired: 10 in]
    n136 = Bundle By Name(cluster=T4 {"仪器编号:"="", "工作状态:"="", "运行量程: "="", "数据时间:"=timestamp(0 s since 1904-01-01), "实测值:"="", "数据标识: "="", "仪器时间:"=timestamp(0 s since 1904-01-01), "告警状态: "="", "故障状态:  "="", "因子编码:"=""} ("运行状态"), "仪器编号:"=w87, "仪器时间:"=w86, "工作状态:"=w84, "告警状态:"=w73, "故障状态:"=w71, "运行量程:"=w82, "数据时间:"=w80, "实测值:"=w79, "数据标识:"=w78, "因子编码:"=w77) -> (→"运行状态":T4)
  }
  n137 = while {
    shift-right: [w325] -> _
    shift-left: u32 0 ("y") -> [w327]
    stop <- FALSE stop-if-true
    # "密码权限"
    n138 = local read "布尔"() -> (w328:bool)
    n139 = local read "一级权限"() -> (w330:bool)
    n140 = local read "二级权限"() -> (w331:bool)
    n141 = local read "一级权限"() -> (w321:bool)
    n142 = local read "二级权限"() -> (w322:bool)
    n143 = local read "输入密码"() -> (w334:u32)
    n144 = Wait (ms)(milliseconds to wait=u32 1000 ("等待时间（毫秒）")) -> ()  [unwired: 1 out]
    n145 = case shown="假" w328 {
      tunnel: w327 -> [_ w340]
      tunnel: [_ w339] -> w325
      frame False {
      }
      frame True {
        n146 = Increment(x=w340) -> (x+1=w339:u32)
      }
    }
    n147 = global read "VAR总磷总氮全局变量.vi" "MB session in"() -> (w320:refnum<class "MB_Master.lvclass">)
    n148 = Or(x=w330, y=w331) -> (x .or. y?=→"布尔":bool)
    n149 = Equal?(x=w334, y=u32 23506) -> (x = y?=→"二级权限":bool)
    n150 = Or(x=w321, y=w322) -> (x .or. y?=w317:bool)
    n151 = Equal?(x=w334, y=u32 666) -> (x = y?=→"一级权限":bool)
    n152 = property class="MB_Master"(reference=w320) -> ("Properties:Session Valid"=w319:bool)  [unwired: 1 in, 2 out]
    n153 = property on="流程固件" class="Bool"("Visible"=w317) -> ()  [unwired: 2 in, 2 out]
    n154 = property on="启动参数设置" class="Bool"("Visible"=w317) -> ()  [unwired: 2 in, 2 out]
    n155 = property on="灯值调整" class="Bool"("Visible"=w317) -> ()  [unwired: 2 in, 2 out]
    n156 = Not(x=w319) -> (.not. x?=w318:bool)
    n157 = Greater Or Equal?(x=w325, y=u32 120) -> (x >= y?=w323:bool)
    n158 = property on="模块启用" class="Bool (严格)"("Value"=w318) -> ()  [unwired: 2 in, 2 out]
    n159 = case shown="假" w323 {
      frame False {
      }
      frame True {
        n160 = local write "输入密码"(u32 0 ("输入密码")) -> ()
      }
    }
  }
  n161 = while {
    shift-right: [w343] -> _
    shift-left: _ -> [w344]
    stop <- FALSE stop-if-true
    n162 = global read "VAR总磷总氮全局变量.vi" "状态告警区"() -> (w341:T7)
    n163 = Wait (ms)(milliseconds to wait=u32 100) -> ()  [unwired: 1 out]
    n164 = Unbundle By Name(w341) -> ("工作状态"=w342:T9, "id"=w348:u16, "日志代码"=w347:u16, "故障代码"=w346:u16, "告警代码"=w345:u16)
    n165 = case shown="\"水样测试\", 默认" w342 {
      tunnel: w348 -> [_ _]
      tunnel: w347 -> [_ w362]
      tunnel: w346 -> [_ w359]
      tunnel: w345 -> [_ w358]
      tunnel: w344 -> [w351 w357]
      tunnel: [w351 w356] -> w343
      frame "空闲" {
      }
      frame "水样测试", Default {
        n166 = call "id参数转换.vi"("id"=u16 1) -> ("table输出"=w360:string)  [unwired: 10 in]
        n167 = Add(x=w359, y=w358) -> (x+y=w356:u16)
        n168 = Not Equal?(x=w356, y=w357) -> (x != y?=w354:bool)
        n169 = Not Equal To 0?(x=w356) -> (x != 0?=w355:bool)
        n170 = call "故障告警分析.vi"("告警代码"=w358, "故障代码"=w359, "运行步序"=w362, "参数"=w360) -> ("报警内容"=w361:T16)  [unwired: 6 in, 1 out]
        n171 = And(x=w355, y=w354) -> (x .and. y?=w353:bool)
        n172 = case shown="真" w353 {
          tunnel: w361 -> [_ w369]
          frame False {
          }
          frame True {
            n173 = Unbundle By Name(w369) -> ("参数"=w365:string, "报警内容"=w364:string, "报警分析"=w363:string)
            n174 = Get Date/Time In Seconds() -> (seconds since 1Jan1904=w368:timestamp)
            n175 = Bundle By Name(cluster=T15 {"时间标识"=timestamp(0 s since 1904-01-01), "设备"="", "日志信息"="", "备注"=""} ("data in"), "时间标识"=w368, "设备"=w365, "日志信息"=w364, "备注"=w363) -> (w367:T15)
            n176 = call "总磷总氮报警信息.vi"("data in"=w367) -> ()  [unwired: 10 in, 1 out]
          }
        }
      }
    }
  }
  n177 = Read from Text File(file (use dialog)=w4) -> (text=w5:string)  [unwired: 3 in, 3 out]
  n178 = while {
    shift-right: [w372] -> _
    shift-left: w5 -> [w374]
    tunnel: w4 -> [w371]
    stop <- FALSE stop-if-true
    n179 = Read from Text File(file (use dialog)=w371) -> (text=w372:string)  [unwired: 3 in, 3 out]
    n180 = Not Equal?(x=w374, y=w372) -> (x != y?=w373:bool)
    n181 = Wait (ms)(milliseconds to wait=u32 1000 ("等待时间（毫秒）")) -> ()  [unwired: 1 out]
    n182 = case shown="真" w373 {
      tunnel: w371 -> [_ w376]
      frame False {
      }
      frame True {
        n183 = vi-ref "总磷总氮断电保存全局变量.vi"() -> (w380:refnum<vi>)
        n184 = call <vilib>:"Open Config Data.vi"("configuration file path"=w376) -> ("error out"=w378:errorcluster, "refnum"=w381:T17)  [unwired: 8 in, 1 out]
        n185 = call <userlib>:"Read Panel from INI__ogtk.vi"("error in (no error)"=w378, "VI ref"=w380, "refnum"=w381) -> ("error out"=w377:errorcluster, "refnum out"=w379:T17)  [unwired: 7 in]
        n186 = call <vilib>:"Close Config Data.vi"("error in (no error)"=w377, "refnum"=w379) -> ()  [unwired: 8 in, 2 out]
      }
    }
  }
  n187 = while {
    tunnel: w10 -> [_]
    stop <- FALSE stop-if-true
    # "试剂填充 172 \n管路清洗108\n氨氮92\n总磷131\n总磷海水147\n总氮76\n总氮海水92"
    n188 = global read "VAR总磷总氮全局变量.vi" "状态告警区"() -> (w408:T7)
    n189 = global read "VAR总磷总氮全局变量.vi" "状态告警区"() -> (w406:T7)
    n190 = global read "VAR总磷总氮全局变量.vi" "状态告警区"() -> (w412:T7)
    n191 = global read "VAR总磷总氮全局变量.vi" "状态告警区"() -> (w404:T7)
    n192 = Wait (ms)(milliseconds to wait=u32 1000 ("等待时间（毫秒）")) -> ()  [unwired: 1 out]
    n193 = Unbundle By Name(w412) -> ("id"=w409:u16, "flowid"=w411:u16, "量程"=w410:u16, "工作状态"=w397:T9, "F0"=→"F0":sgl, "F1"=→"F1":sgl, "F2"=→"F2":sgl, "F3"=→"F3":sgl, "ADC"=→"ADC":sgl, "总磷控温温度1"=→"温度1":sgl, "营养盐控温温度2"=→"温度2":sgl)
    n194 = Unbundle By Name(w404) -> ("日志代码"=w403:u16)
    n195 = Unbundle By Name(w408) -> ("日志代码"=w400:u16)
    n196 = Unbundle By Name(w406) -> ("工作状态"=w392:T9, "id"=w393:u16)
    n197 = case shown="\"空闲\"" w392 {
      frame "空闲" {
        n198 = local write "数组"(string[] [] ("数组")) -> ()
      }
      frame "水样测试", Default {
      }
    }
    n199 = feedback-in #2(w400) -> ()
    n200 = feedback #2(w400) -> (w417:u16)
    n201 = feedback #3(w403) -> (w405:u16)
    n202 = feedback-in #3(w403) -> ()
    n203 = Not Equal To 0?(x=w392) -> (x != 0?=w390:bool)
    n204 = Subtract(x=w400, y=1) -> (x-y=→"多列列表框":i32)
    n205 = Not Equal?(x=w400, y=w417) -> (x != y?=w416:bool)
    n206 = call <vilib>:"Boolean Crossing PtByPt.vi"("direction"=enum16{"either", "false-true", "true-false"}."false-true", "input"=w390) -> ("crossing"=w394:bool)  [unwired: 1 in]
    n207 = call <vilib>:"Boolean Crossing PtByPt.vi"("direction"=enum16{"either", "false-true", "true-false"}."true-false", "input"=w390) -> ("crossing"=w389:bool)  [unwired: 1 in]
    n208 = Not Equal To 0?(x=w397) -> (x != 0?=w414:bool)
    n209 = case shown="假" w416 {
      tunnel: w400 -> [_ w553]
      frame False {
      }
      frame True {
        n210 = Subtract(x=w553, y=1) -> (x-y=w551:i32)
        n211 = Subtract(x=w551, y=5) -> (x-y=w555:i32)
        n212 = Greater Or Equal To 0?(x=w555) -> (x >= 0?=w554:bool)
        n213 = property on="多列列表框" class="MCListbox (严格)"() -> (error out=w559:errorcluster, "TopLeft"=w560:T20)  [unwired: 2 in, 1 out]
        n214 = Select(t=w555, s=w554, f=0) -> (s? t:f=w556:i32)
        n215 = Bundle By Name(cluster=w560, "Row"=w556) -> (w561:T20)
        n216 = property on="多列列表框" class="MCListbox (严格)"(error in=w559, "TopLeft"=w561) -> ()  [unwired: 1 in, 2 out]
      }
    }
    n217 = case shown="真" w394 {
      tunnel: w392 -> [_ w443]
      tunnel: w393 -> [_ w440]
      frame False {
      }
      frame True {
        n218 = case shown="\"空闲\", 默认" w443 {
          tunnel: [_ "【水样测试】" ("字符串") "【标样核查】" ("字符串") "【零点核查】" ("字符串") "【跨度核查】" ("字符串") "【空白测试】" ("字符串") "【平行样测试】" ("字符串") "【加标回收】" ("字符串") "【空白校准】" ("字符串") "【标样校准】" ("字符串")] -> w448
          frame "空闲", Default {
          }
          frame "水样测试" {
          }
          frame "标样核查" {
          }
          frame "零点核查" {
          }
          frame "跨度核查" {
          }
          frame "空白测试" {
          }
          frame "平行样测试" {
          }
          frame "加标回收" {
          }
          frame "空白校准" {
          }
          frame "标样校准" {
          }
        }
        n219 = call "id参数转换.vi"("id"=w440) -> ("table输出"=w439:string)  [unwired: 10 in]
        n220 = Concatenate Strings("-->>" ("字符串"), w448, "启动" ("字符串")) -> (w447:string)
        n221 = Get Date/Time In Seconds() -> (seconds since 1Jan1904=w445:timestamp)
        n222 = Bundle By Name(cluster=T19 {"时间标识"=timestamp(0 s since 1904-01-01), "设备"="", "日志信息"="", "流程参数"=""} ("data in"), "时间标识"=w445, "设备"=w439, "日志信息"=w447) -> (w444:T19)
        n223 = call "总磷总氮操作日志.vi"("data in"=w444) -> ()  [unwired: 11 in]
      }
    }
    n224 = case shown="真" w389 {
      tunnel: w392 -> [_ w424]
      tunnel: w393 -> [_ w421]
      frame False {
      }
      frame True {
        n225 = case shown="\"水样测试\"" w424 {
          tunnel: [_ "【水样测试】" ("字符串") "【标样核查】" ("字符串") "【零点核查】" ("字符串") "【跨度核查】" ("字符串") "【空白测试】" ("字符串") "【平行样测试】" ("字符串") "【加标回收】" ("字符串") "【空白校准】" ("字符串") "【标样校准】" ("字符串")] -> w429
          frame "空闲", Default {
          }
          frame "水样测试" {
          }
          frame "标样核查" {
          }
          frame "零点核查" {
          }
          frame "跨度核查" {
          }
          frame "空白测试" {
          }
          frame "平行样测试" {
          }
          frame "加标回收" {
          }
          frame "空白校准" {
          }
          frame "标样校准" {
          }
        }
        n226 = call "id参数转换.vi"("id"=w421) -> ("table输出"=w420:string)  [unwired: 10 in]
        n227 = Concatenate Strings("-->>" ("字符串"), w429, "停止" ("字符串")) -> (w428:string)
        n228 = Get Date/Time In Seconds() -> (seconds since 1Jan1904=w426:timestamp)
        n229 = Bundle By Name(cluster=T19 {"时间标识"=timestamp(0 s since 1904-01-01), "设备"="", "日志信息"="", "流程参数"=""} ("data in"), "时间标识"=w426, "设备"=w420, "日志信息"=w428) -> (w425:T19)
        n230 = call "总磷总氮操作日志.vi"("data in"=w425) -> ()  [unwired: 11 in]
      }
    }
    n231 = call <vilib>:"Boolean Crossing PtByPt.vi"("input"=w414) -> ("crossing"=w396:bool)  [unwired: 2 in]
    n232 = Bundle By Name(cluster=T18 {"启动模式"=enum."跨度核查", "启动参数"=1, "量程"=enum."低量程"} ("参数簇"), "启动参数"=w409, "启动模式"=w411, "量程"=w410) -> (w407:T18)
    n233 = First Call?() -> (First Call?: T/F=w415:bool)
    n234 = Or(x=w396, y=w415) -> (x .or. y?=w413:bool)
    n235 = while {
      tunnel: w413 -> [w539]
      tunnel: w407 -> [w538]
      shift-right: [w533] -> _
      shift-left: _ -> [w535]
      shift-right: [w534] -> _
      shift-left: _ -> [w536]
      shift-right: ["流程路径"] -> _
      shift-left: _ -> [w531]
      stop <- TRUE stop-if-true
      n236 = Not Equal?(x=w531, y="流程路径") -> (x != y?=w529:bool)
      n237 = Or(x=w539, y=w529) -> (x .or. y?=w530:bool)
      n238 = case shown="真" w530 {
        tunnel: [w541 w549] -> w534
        tunnel: [w540 w548] -> w533
        tunnel: w538 -> [_ w543]
        tunnel: w536 -> [w541 _]
        tunnel: w535 -> [w540 _]
        tunnel: "流程路径" -> [_ w542]
        frame False {
        }
        frame True {
          n239 = call "斯坦道XML解析.vi"("添加的路径"=w542, "参数簇"=w543) -> ("步骤时间"=w544:string[], "步骤名"=w546:string[])  [unwired: 8 in]
          n240 = Build Array(w546, w544) -> (w545:string[][])
          n241 = for {
            tunnel: w546 -> [_] mode=indexing
            tunnel: [w550] -> w547 mode=indexing
            i -> [w550]
          }
          n242 = Transpose 2D Array(2D array=w545) -> (transposed array=w548:string[][])
          n243 = Number To Decimal String(number=w547) -> (decimal integer string=w549:string[])  [unwired: 1 in]
        }
      }
      n244 = property on="多列列表框" class="MCListbox (严格)"("ItemNames"=w533, "RowHdrs[]"=w534) -> ()  [unwired: 2 in, 2 out]
    }
    n245 = Not Equal?(x=w403, y=w405) -> (x != y?=w402:bool)
    n246 = case shown="真" w402 {
      frame False {
      }
      frame True {
        n247 = property on="多列列表框" class="MCListbox (严格)"() -> ("ItemNames"=w463:string[][], "Value"=w459:i32)  [unwired: 2 in, 2 out]
        n248 = Index Array(array=w463, index (row)=w459) -> (element=w462:string[])  [unwired: 1 in]
        n249 = Index Array(array=w462) -> (element=w461:string)  [unwired: 1 in]
        n250 = call "过滤筛选流程.vi"("字符串"=w461) -> ("匹配后偏移量"=w460:i32)  [unwired: 10 in]
        n251 = case shown="默认" w460 {
          tunnel: w461 -> [w465 _]
          tunnel: w459 -> [w464 _]
          frame Default {
            n252 = case shown="默认" w465 {
              selector: w465 -> [w471 w478]
              tunnel: [w471 w478] -> w467
              tunnel: [string[] [] ("数组") w473] -> w466
              tunnel: w464 -> [_ w477]
              frame "读数" {
              }
              frame Default {
                n253 = Equal?(x=w477, y=1) -> (x = y?=w475:bool)
                n254 = Select(t=string[] [], s=w475, f="数组") -> (s? t:f=w473:string[])
              }
            }
            n255 = for {
              N: 1 -> [_]
              tunnel: w467 -> [w480]
              shift-right: [w479] -> w468
              shift-left: w466 -> [w481]
              n256 = Search 1D Array(1D array=w481, element=w480) -> (index of element=w484:i32)  [unwired: 1 in]
              n257 = Format Into String(format string="%s" ("格式字符串"), w480) -> (resulting string=w485:string)  [unwired: 2 in, 1 out]
              n258 = Equal?(x=w484, y=-1) -> (x = y?=w482:bool)
              n259 = case shown="真" w482 {
                tunnel: w485 -> [_ w495]
                tunnel: w481 -> [w487 w499]
                tunnel: w480 -> [_ w498]
                tunnel: [w487 w497] -> w479
                frame False {
                }
                frame True {
                  n260 = case shown="\"结束\"" w495 {
                    selector: w495 -> [w522 w525 w528]
                    tunnel: [w522 w524 w527] -> w494
                    frame Default {
                    }
                    frame "初始化" {
                      n261 = Concatenate Strings("-->>" ("字符串"), w525) -> (w524:string)
                    }
                    frame "结束" {
                      n262 = Concatenate Strings("-->>" ("字符串"), w528) -> (w527:string)
                    }
                  }
                  n263 = Insert Into Array(array=w499, new element=w498) -> (w497:string[])  [unwired: 1 in]
                  n264 = global read "VAR总磷总氮全局变量.vi" "状态告警区"() -> (w493:T7)
                  n265 = Unbundle By Name(w493) -> ("工作状态"=w492:T9)
                  n266 = case shown="\"水样测试\"" w492 {
                    tunnel: [_ "【水样测试】" ("字符串") "【标样核查】" ("字符串") "【零点核查】" ("字符串") "【跨度核查】" ("字符串") "【空白测试】" ("字符串") "【平行样测试】" ("字符串") "【加标回收】" ("字符串") "【空白校准】" ("字符串") "【标样校准】" ("字符串")] -> w490
                    frame "空闲", Default {
                    }
                    frame "水样测试" {
                    }
                    frame "标样核查" {
                    }
                    frame "零点核查" {
                    }
                    frame "跨度核查" {
                    }
                    frame "空白测试" {
                    }
                    frame "平行样测试" {
                    }
                    frame "加标回收" {
                    }
                    frame "空白校准" {
                    }
                    frame "标样校准" {
                    }
                  }
                  n267 = global read "VAR总磷总氮全局变量.vi" "状态告警区"() -> (w512:T7)
                  n268 = global read "VAR总磷总氮全局变量.vi" "状态告警区"() -> (w509:T7)
                  n269 = Unbundle By Name(w509) -> ("F0"=w506:sgl, "F1"=w505:sgl, "F2"=w504:sgl, "F3"=w503:sgl, "id"=w502:u16, "flowid"=w501:u16, "量程"=w500:u16)
                  n270 = Unbundle By Name(w512) -> ("id"=w489:u16)
                  n271 = call "id参数转换.vi"("id"=w489) -> ("table输出"=w488:string)  [unwired: 10 in]
                  n272 = Concatenate Strings(w490, w494) -> (w491:string)
                  n273 = Format Into String(format string="F0=%#f,F1=%#f,F2=%#f,F3=%#f,Flow=%d-%-d-%-d" ("格式字符串"), w506, w505, w504, w503, w502, w501, w500) -> (resulting string=w507:string)  [unwired: 2 in, 1 out]
                  n274 = Get Date/Time In Seconds() -> (seconds since 1Jan1904=w510:timestamp)
                  n275 = Bundle By Name(cluster=T19 {"时间标识"=timestamp(0 s since 1904-01-01), "设备"="", "日志信息"="", "流程参数"=""} ("data in"), "时间标识"=w510, "设备"=w488, "日志信息"=w491, "流程参数"=w507) -> (w511:T19)
                  n276 = call "总磷总氮操作日志.vi"("data in"=w511) -> ()  [unwired: 11 in]
                }
              }
            }
            n277 = local write "数组"(w468) -> ()
          }
          frame -1 {
          }
        }
      }
    }
  }
  n278 = flat-sequence {
    tunnel: [w577] -> w6
    frame #0 {
      n279 = call "配置文件路径.vi"() -> ("appended path"=w570:path)  [unwired: 11 in]
      n280 = control-ref of="本VI"() -> (w569:refnum<vi>)
      n281 = call <vilib>:"Open Config Data.vi"("configuration file path"=w570) -> ("error out"=w574:errorcluster, "refnum"=w571:T17)  [unwired: 8 in, 1 out]
      n282 = property class="VI"(reference=w569) -> ("Library.Version"=w568:T21)  [unwired: 1 in, 2 out]
      n283 = vi-ref "总磷总氮断电保存全局变量.vi"() -> (w572:refnum<vi>)
      n284 = Unbundle By Name(w568) -> ("Major"=w566:u16, "Minor"=w565:u16, "Fix"=w564:u16, "Build"=w563:u16)
      n285 = call <userlib>:"Read Panel from INI__ogtk.vi"("error in (no error)"=w574, "VI ref"=w572, "refnum"=w571) -> ("error out"=w575:errorcluster, "refnum out"=w573:T17)  [unwired: 7 in]
      n286 = call <vilib>:"Close Config Data.vi"("error in (no error)"=w575, "refnum"=w573) -> ()  [unwired: 8 in, 2 out]
      n287 = Format Into String(format string="模块版本号：%d.%d.%d.%d" ("格式字符串"), w566, w565, w564, w563) -> (resulting string=→"模块版本号":string)  [unwired: 2 in, 1 out]
    }
    frame #1 {
      n288 = control-ref of="本VI"() -> (w578:refnum<vi>)
      n289 = vi-ref "总磷总氮通讯.vi"() -> (w593:refnum<vi>)
      n290 = global read "总磷总氮断电保存全局变量.vi" "启动参数"() -> (w581:T12)
      n291 = property class="VI"(reference=w578) -> ("Library"=w579:refnum<vi>)  [unwired: 1 in, 2 out]
      n292 = property class="Library"(reference=w579) -> ("LocalName"=w580:string)  [unwired: 1 in, 2 out]
      n293 = Cluster To Array(cluster=w581) -> (array=w582:bool[])
      n294 = vi-ref "总磷总氮测量数据储存.vi"() -> (w601:refnum<vi>)
      n295 = property class="VI"(reference=w593) -> ("Name"=w594:string)  [unwired: 1 in, 2 out]
      n296 = vi-ref "关键参数交互.vi"() -> (w592:refnum<vi>)
      n297 = property on="定时设置" class="定时设置 (严格)"("引用参数"=w580) -> ()  [unwired: 2 in, 2 out]
      n298 = for {
        tunnel: w582 -> [w609] mode=indexing
        tunnel: [w610] -> w584 mode=indexing if=w611
        tunnel: [w610] -> w583 mode=indexing if=w609
        i -> [w610]
        n299 = Not(x=w609) -> (.not. x?=w611:bool)
      }
      n300 = property class="VI"(reference=w601) -> ("Name"=w608:string)  [unwired: 1 in, 2 out]
      n301 = Open VI Reference(type specifier VI Refnum (for type only)=refnum<vi> refnum, vi path=w594, options=128 ("选项")) -> (vi reference=w596:refnum<vi>, error out=w598:errorcluster)  [unwired: 3 in]
      n302 = property class="VI"(reference=w592) -> ("Name"=w586:string)  [unwired: 1 in, 2 out]
      n303 = call-by-ref "开始异步调用"(reference=w596, error in=w598) -> (reference out=w600:refnum<vi>, error out=w599:errorcluster)  [unwired: 12 in]
      n304 = Open VI Reference(type specifier VI Refnum (for type only)=refnum<vi> refnum, vi path=w608, options=128 ("选项")) -> (vi reference=w606:refnum<vi>, error out=w604:errorcluster)  [unwired: 3 in]
      n305 = Close Reference(reference=w600, error in (no error)=w599) -> ()  [unwired: 1 out]
      n306 = Index Array(array=w583) -> (element=w576:i32)  [unwired: 1 in]
      n307 = Open VI Reference(type specifier VI Refnum (for type only)=refnum<vi> refnum, vi path=w586, options=128 ("选项")) -> (vi reference=w588:refnum<vi>, error out=w589:errorcluster)  [unwired: 3 in]
      n308 = property on="参数下拉列表" class="Enum (严格)"("Disabled Items []"=w584, "Val(Sgnl)"=w576) -> ()  [unwired: 2 in, 2 out]
      n309 = call-by-ref "开始异步调用"(reference=w606, error in=w604) -> (reference out=w602:refnum<vi>, error out=w603:errorcluster)  [unwired: 12 in]
      n310 = Close Reference(reference=w602, error in (no error)=w603) -> ()  [unwired: 1 out]
      n311 = call-by-ref "开始异步调用"(reference=w588, error in=w589) -> (reference out=w591:refnum<vi>, error out=w590:errorcluster)  [unwired: 12 in]
      n312 = Close Reference(reference=w591, error in (no error)=w590) -> ()  [unwired: 1 out]
      n313 = call "设置模块队列名.vi"() -> ("Msg"=w577:string)  [unwired: 5 in]
    }
  }
  n314 = Obtain Queue(name (unnamed)=w6, element data type=cluster{"命令":string, "data":variant} {"命令"="", "data"=variant}) -> (queue out=w7:refnum<queue>)  [unwired: 3 in, 2 out]
  n315 = control-ref of="测量模式下拉列表"() -> (w13:refnum<vi>)
  n316 = while {
    tunnel: w7 -> [w616]
    tunnel: [w614] -> _
    stop <- FALSE stop-if-true
    # "定时更新"
    n317 = Get Queue Status(queue=w616) -> (queue out=w613:refnum<queue>, # elements in queue=w612:i32)  [unwired: 2 in, 6 out]
    n318 = Wait (ms)(milliseconds to wait=u32 1000 ("等待时间（毫秒）")) -> ()  [unwired: 1 out]
    n319 = case shown="0" w612 {
      tunnel: w613 -> [_ w624]
      tunnel: [_ w622] -> w614
      frame Default {
      }
      frame 0 {
        n320 = global read "VAR总磷总氮全局变量.vi" "启动队列名称"() -> (w620:cluster{"String":string, "Value":u16}[])
        n321 = Index Array(array=w620) -> (element=w619:cluster{"String":string, "Value":u16})  [unwired: 1 in]
        n322 = Unbundle By Name(w619) -> ("Value"=w618:u16)
        n323 = call "总磷总氮版本号读取.vi"("Slave ID"=w618) -> ("error out"=w622:errorcluster, "固件版本号"=→"固件版本号":string)  [unwired: 9 in]
        n324 = Bundle By Name(cluster=cluster{"命令":string, "data":variant} {"命令"="", "data"=variant} ("元素"), "命令"="读序列号", "data"=w618) -> (w623:cluster{"命令":string, "data":variant})
        n325 = Enqueue Element(queue=w624, element=w623) -> ()  [unwired: 2 in, 3 out]
      }
    }
  }
  n326 = while {
    tunnel: w7 -> [w632]
    stop <- FALSE stop-if-true
    n327 = Get Queue Status(queue=w632) -> (queue out=w630:refnum<queue>, # elements in queue=w629:i32)  [unwired: 2 in, 6 out]
    n328 = Wait (ms)(milliseconds to wait=u32 1000 ("等待时间（毫秒）")) -> ()  [unwired: 1 out]
    n329 = case shown="0" w629 {
      tunnel: w630 -> [_ w648]
      frame Default {
      }
      frame 0 {
        n330 = global read "VAR总磷总氮全局变量.vi" "启动队列名称"() -> (w637:cluster{"String":string, "Value":u16}[])
        n331 = for {
          tunnel: [w666] -> w638 mode=indexing
          tunnel: w637 -> [w667] mode=indexing
          n332 = Unbundle By Name(w667) -> ("Value"=w666:u16)
        }
        n333 = global read "VAR总磷总氮全局变量.vi" "状态告警区"() -> (w640:T7)
        n334 = Unbundle By Name(w640) -> ("系统时间"=w647:timestamp, "工作状态"=w639:T9)
        n335 = for {
          tunnel: w639 -> [w652]
          shift-right: [w653] -> w641
          shift-left: w648 -> [w655]
          tunnel: w638 -> [w649] mode=indexing
          n336 = Equal?(x=w652, y=T9."空闲") -> (x = y?=w650:bool)
          n337 = Bundle By Name(cluster=cluster{"命令":string, "data":variant} {"命令"="", "data"=variant} ("元素"), "命令"="读状态告警区", "data"=w649) -> (w657:cluster{"命令":string, "data":variant})
          n338 = Enqueue Element(queue=w655, element=w657) -> (queue out=w654:refnum<queue>)  [unwired: 2 in, 2 out]
          n339 = case shown="真" w650 {
            tunnel: w654 -> [w659 w662]
            tunnel: w649 -> [_ w661]
            tunnel: [w659 w660] -> w653
            frame False {
            }
            frame True {
              n340 = Bundle By Name(cluster=cluster{"命令":string, "data":variant} {"命令"="", "data"=variant} ("元素"), "命令"="读测量数据区", "data"=w661) -> (w664:cluster{"命令":string, "data":variant})
              n341 = Enqueue Element(queue=w662, element=w664) -> (queue out=w660:refnum<queue>)  [unwired: 2 in, 2 out]
            }
          }
        }
        n342 = Get Date/Time In Seconds() -> (seconds since 1Jan1904=w646:timestamp)
        n343 = Subtract(x=w646, y=w647) -> (x-y=w645:dbl)
        n344 = Absolute Value(x=w645) -> (abs(x)=w644:dbl)
        n345 = Greater Or Equal?(x=w644, y=120.0) -> (x >= y?=w642:bool)
        n346 = case shown="真" w642 {
          tunnel: w641 -> [_ w669]
          frame False {
          }
          frame True {
            n347 = call "总磷总氮启动命令.vi"("参数"=T22 {"站号"=3, "量程切换"=enum."AUTO", "控制命令"=enum."校时", "模式设置"=enum."待机", "测量间隔"=0}) -> ("启动命令"=w668:cluster{"命令":string, "data":variant})  [unwired: 10 in]
            n348 = Enqueue Element(queue=w669, element=w668) -> ()  [unwired: 2 in, 3 out]
          }
        }
      }
    }
    n349 = global read "总磷总氮断电保存全局变量.vi" "流程路径"() -> (w631:path)
    n350 = global read "总磷总氮断电保存全局变量.vi" "MB通信方式选择"() -> (w628:enum16{"串口", "TCP"})
    n351 = local write "流程路径"(w631) -> ()
    n352 = case shown="\"串口\", 默认" w628 {
      tunnel: [w635 w636] -> w627
      frame "串口", Default {
        n353 = global read "总磷总氮断电保存全局变量.vi" "VISA Resource"() -> (w635:refnum<visa-resource-name>)
      }
      frame "TCP" {
        n354 = global read "总磷总氮断电保存全局变量.vi" "IP"() -> (w636:string)
      }
    }
    "字符串 2" <- w627
  }
  n355 = call "设置模块队列名.vi"() -> ("Msg"=w2:string)  [unwired: 5 in]
  n356 = control-ref of="量程参数读取"() -> (w11:refnum<vi>)
  n357 = control-ref of="参数下拉列表"() -> (w14:refnum<vi>)
  n358 = control-ref of="量程下拉列表"() -> (w15:refnum<vi>)
  n359 = control-ref of="公式"() -> (w12:refnum<vi>)
  n360 = Obtain Notifier(name (unnamed)=w2, notification data type=FALSE) -> (notifier out=w1:refnum<notifier>)  [unwired: 2 in, 2 out]
  n361 = while {
    tunnel: w7 -> [w677]
    tunnel: w15 -> [w676]
    tunnel: w14 -> [w675]
    tunnel: w13 -> [w674]
    tunnel: w12 -> [w673]
    tunnel: w11 -> [w672]
    tunnel: w1 -> [w671]
    stop <- FALSE stop-if-true
    n362 = event shown="[4] \"测量模式下拉列表\", \"量程下拉列表\", \"参数下拉列表\": 值改变" {
      selector: _ -> [_ _ _ _ _ _ _ _ _ _ _ _ _ _ _ _ _ _ _ _ _ _ _ _]
      dyn-events: _ -> [_ _ _ _ _ _ _ _ _ _ _ _ _ _ _ _ _ _ _ _ _ _ _ _]
      timeout: _ -> [_ _ _ _ _ _ _ _ _ _ _ _ _ _ _ _ _ _ _ _ _ _ _ _]
      tunnel: w677 -> [_ _ _ _ _ _ w697 w723 _ _ _ _ _ _ w820 _ w829 _ _ _ _ _ _ _]
      tunnel: w676 -> [_ _ _ _ _ _ _ _ _ w743 _ _ _ _ _ _ _ _ _ _ w845 _ _ _]
      tunnel: w675 -> [_ _ _ _ _ _ _ _ _ w747 _ _ _ w798 _ _ _ _ _ _ w843 _ w896 w903]
      tunnel: w674 -> [_ _ _ _ _ _ _ _ _ w745 _ _ _ _ _ _ _ _ _ _ w844 _ _ _]
      tunnel: w673 -> [_ _ _ _ _ _ _ _ _ _ _ _ _ _ _ _ _ _ _ _ w839 _ _ _]
      tunnel: w672 -> [_ _ _ _ _ _ _ _ _ _ _ _ _ _ _ _ _ _ _ _ _ _ w894 _]
      tunnel: [_ _ _ _ w683 _ _ _ _ _ _ _ _ _ _ _ _ _ _ _ _ _ _ _] -> _
      tunnel: w671 -> [_ _ _ _ _ _ _ _ _ _ _ _ _ _ _ _ w825 _ _ _ _ _ _ _]
      event Timeout {
        n363 = event-data() -> ()  [unwired: 1 in, 3 out]
      }
      event "灯值调整": Value Change {
        n364 = event-data() -> ()  [unwired: 1 in, 6 out]
        n365 = call "灯值调整对话框.vi"() -> ()  [unwired: 12 in]
      }
      event "启动参数设置": Value Change {
        n366 = event-data() -> ()  [unwired: 1 in, 6 out]
        n367 = call "启动参数设置.vi"() -> ()  [unwired: 12 in]
      }
      event "布尔": Mouse Down {
        n368 = event-data() -> ("CtlRef"=w680:refnum<vi>)  [unwired: 1 in, 5 out]
        n369 = property class="Bool (严格)"(reference=w680) -> ("Value"=w679:bool)  [unwired: 1 in, 2 out]
        n370 = case shown="真" w679 {
          frame False {
            n371 = call "密码键盘.vi"() -> ("NewNumber"=→"输入密码":dbl)  [unwired: 1 in]
          }
          frame True {
            n372 = local write "输入密码"(u32 0 ("输入密码")) -> ()
          }
        }
      }
      event "测量模式下拉列表", "量程下拉列表", "参数下拉列表": Value Change {
        n373 = event-data() -> ()  [unwired: 1 in, 6 out]
        n374 = local read "测量模式下拉列表"() -> (w686:enum16{"水样测量", "零点核查", "跨度核查", "标样核查", "加标回收"})
        n375 = local read "参数下拉列表"() -> (w685:enum16{"COD", "氨氮", "总氮", "总磷"})
        n376 = local read "量程下拉列表"() -> (w687:enum16{"低量程", "高量程"})
        n377 = Bundle("参数下拉列表"=w685, "测量模式下拉列表"=w686, "量程下拉列表"=w687) -> (w684:T23)  [unwired: 1 in]
        n378 = property on="曲线模型" class="曲线模型 (严格)"("属性"=w684) -> (error out=w683:errorcluster)  [unwired: 2 in, 1 out]
      }
      event "流程固件": Value Change {
        n379 = event-data() -> ()  [unwired: 1 in, 6 out]
        n380 = call "流程固件设置对话框.vi"() -> ()  [unwired: 12 in]
      }
      event "串口设置": Value Change {
        n381 = event-data() -> ()  [unwired: 1 in, 6 out]
        n382 = global read "总磷总氮断电保存全局变量.vi" "MB通信方式选择"() -> (w688:enum16{"串口", "TCP"})
        n383 = global read "总磷总氮断电保存全局变量.vi" "VISA Resource"() -> (w694:refnum<visa-resource-name>)
        n384 = global read "总磷总氮断电保存全局变量.vi" "PORT"() -> (w692:string)
        n385 = global read "总磷总氮断电保存全局变量.vi" "IP"() -> (w693:string)
        n386 = call "串口配置.vi"("PORT"=w692, "IP"=w693, "MB通信方式选择"=w688, "请选择串口:"=w694) -> ("PORT 2"=w690:string, "IP 2"=w691:string, "确认 2"=w695:bool, "VISA资源名称 2"=w696:refnum<visa-resource-name>, "MB通信方式选择 2"=w689:enum16{"串口", "TCP"})  [unwired: 3 in]
        n387 = case shown="真" w695 {
          tunnel: w696 -> [_ w702]
          tunnel: w697 -> [_ w701]
          tunnel: w691 -> [_ w700]
          tunnel: w690 -> [_ w699]
          tunnel: w689 -> [_ w698]
          frame False {
          }
          frame True {
            n388 = flat-sequence {
              tunnel: w702 -> [w707]
              tunnel: w701 -> [w708]
              tunnel: w700 -> [w706]
              tunnel: w699 -> [w705]
              tunnel: w698 -> [w704]
              frame #0 {
                n389 = global write "总磷总氮断电保存全局变量.vi" "IP"(w706) -> ()
                n390 = global write "总磷总氮断电保存全局变量.vi" "PORT"(w705) -> ()
                n391 = global write "总磷总氮断电保存全局变量.vi" "VISA Resource"(w707) -> ()
                n392 = global write "总磷总氮断电保存全局变量.vi" "MB通信方式选择"(w704) -> ()
                n393 = Flush Queue(queue=w708) -> (queue out=w703:refnum<queue>)  [unwired: 1 in, 2 out]
                n394 = Enqueue Element(queue=w703, element=cluster{"命令":string, "data":variant} {"命令"="启用模块", "data"=variant} ("元素")) -> ()  [unwired: 2 in, 3 out]
              }
              frame #1 {
                n395 = call "配置文件路径.vi"() -> ("appended path"=w710:path)  [unwired: 11 in]
                n396 = call <vilib>:"Open Config Data.vi"("configuration file path"=w710) -> ("error out"=w718:errorcluster, "refnum"=w721:T17)  [unwired: 8 in, 1 out]
                n397 = vi-ref "总磷总氮断电保存全局变量.vi"() -> (w720:refnum<vi>)
                n398 = call <userlib>:"Write Panel to INI__ogtk.vi"("error in (no error)"=w718, "VI ref"=w720, "refnum"=w721) -> ("error out"=w717:errorcluster, "refnum out"=w719:T17)  [unwired: 7 in]
                n399 = call <vilib>:"Close Config Data.vi"("error in (no error)"=w717, "refnum"=w719) -> ("error out"=w712:errorcluster, "file path"=w711:path)  [unwired: 8 in]
                n400 = Open/Create/Replace File(file path (use dialog)=w711, error in=w712) -> (refnum out=w715:refnum<file>, error out=w716:errorcluster)  [unwired: 4 in, 1 out]
                n401 = Flush File(refnum=w715, error in=w716) -> (refnum out=w714:refnum<file>, error out=w713:errorcluster)
                n402 = Close File(refnum=w714, error in=w713) -> ()  [unwired: 2 out]
              }
            }
          }
        }
      }
      event "模块启用": Value Change {
        n403 = event-data() -> ("OldVal"=w724:bool)  [unwired: 1 in, 5 out]
        n404 = Flush Queue(queue=w723) -> (queue out=w722:refnum<queue>)  [unwired: 1 in, 2 out]
        n405 = case shown="假" w724 {
          tunnel: w722 -> [w725 w727]
          frame False {
            n406 = Enqueue Element(queue=w725, element=cluster{"命令":string, "data":variant} {"命令"="停用模块", "data"=variant} ("元素")) -> ()  [unwired: 2 in, 3 out]
          }
          frame True {
            n407 = Enqueue Element(queue=w727, element=cluster{"命令":string, "data":variant} {"命令"="启用模块", "data"=variant} ("元素")) -> ()  [unwired: 2 in, 3 out]
          }
        }
      }
      event "流程路径": Value Change {
        n408 = event-data() -> ()  [unwired: 1 in, 6 out]
        n409 = flat-sequence {
          frame #0 {
            n410 = local read "流程路径"() -> (w729:path)
            n411 = global write "总磷总氮断电保存全局变量.vi" "流程路径"(w729) -> ()
          }
          frame #1 {
            n412 = call "配置文件路径.vi"() -> ("appended path"=w730:path)  [unwired: 11 in]
            n413 = call <vilib>:"Open Config Data.vi"("configuration file path"=w730) -> ("error out"=w738:errorcluster, "refnum"=w741:T17)  [unwired: 8 in, 1 out]
            n414 = vi-ref "总磷总氮断电保存全局变量.vi"() -> (w740:refnum<vi>)
            n415 = call <userlib>:"Write Panel to INI__ogtk.vi"("error in (no error)"=w738, "VI ref"=w740, "refnum"=w741) -> ("error out"=w737:errorcluster, "refnum out"=w739:T17)  [unwired: 7 in]
            n416 = call <vilib>:"Close Config Data.vi"("error in (no error)"=w737, "refnum"=w739) -> ("error out"=w732:errorcluster, "file path"=w731:path)  [unwired: 8 in]
            n417 = Open/Create/Replace File(file path (use dialog)=w731, error in=w732) -> (refnum out=w735:refnum<file>, error out=w736:errorcluster)  [unwired: 4 in, 1 out]
            n418 = Flush File(refnum=w735, error in=w736) -> (refnum out=w734:refnum<file>, error out=w733:errorcluster)
            n419 = Close File(refnum=w734, error in=w733) -> ()  [unwired: 2 out]
          }
        }
      }
      event "公式一键写入": Value Change {
        n420 = event-data() -> ()  [unwired: 1 in, 6 out]
        n421 = property class="Enum (严格)"(reference=w747) -> ("Value"=w746:enum16{"COD", "氨氮", "总氮", "总磷"})  [unwired: 1 in, 2 out]
        n422 = property class="Enum (严格)"(reference=w745) -> ("Value"=w744:enum16{"水样测量", "零点核查", "跨度核查", "标样核查", "加标回收"})  [unwired: 1 in, 2 out]
        n423 = property class="Enum (严格)"(reference=w743) -> ("Value"=w742:enum16{"低量程", "高量程"})  [unwired: 1 in, 2 out]
        n424 = local read "公式"() -> (w749:cluster{"X^2":dbl, "X":dbl, "b":dbl})
        n425 = call "公式复合写入.vi"("公式"=w749, "量程下拉列表"=w742, "测量模式下拉列表"=w744, "参数下拉列表"=w746) -> ("模型复制"=w748:T24)  [unwired: 7 in]
        n426 = invoke on="曲线模型" class="曲线模型 (严格)" method="模型复制.vi"("模型复制"=w748) -> ()  [unwired: 3 in, 4 out]
      }
      event "曲线模型": Value Change {
        n427 = event-data() -> ()  [unwired: 1 in, 6 out]
        n428 = Unbundle By Name("曲线模型") -> ("X^2"=w753:dbl, "X"=w752:dbl, "B"=w751:dbl)
        n429 = Bundle("X^2"=w753, "X"=w752, "B"=w751) -> (w750:cluster{"X^2":dbl, "X":dbl, "B":dbl})  [unwired: 1 in]
        n430 = local write "公式"(w750) -> ()
      }
      event "质控参数设置": Value Change {
        n431 = event-data() -> ()  [unwired: 1 in, 6 out]
        n432 = global read "总磷总氮断电保存全局变量.vi" "质控参数设置"() -> (w757:T25)
        n433 = call "总磷总氮质控参数设置.vi"("质控参数设置"=w757) -> ("质控参数设置 2"=w755:T25, "check？"=w756:bool)  [unwired: 9 in]
        n434 = case shown="真" w756 {
          tunnel: w757 -> [_ w759]
          tunnel: w755 -> [_ w758]
          frame False {
          }
          frame True {
            n435 = flat-sequence {
              tunnel: w759 -> [_]
              tunnel: w758 -> [w760]
              frame #0 {
                n436 = global write "总磷总氮断电保存全局变量.vi" "质控参数设置"(w760) -> ()
              }
              frame #1 {
                n437 = call "配置文件路径.vi"() -> ("appended path"=w761:path)  [unwired: 11 in]
                n438 = call <vilib>:"Open Config Data.vi"("configuration file path"=w761) -> ("error out"=w769:errorcluster, "refnum"=w772:T17)  [unwired: 8 in, 1 out]
                n439 = vi-ref "总磷总氮断电保存全局变量.vi"() -> (w771:refnum<vi>)
                n440 = call <userlib>:"Write Panel to INI__ogtk.vi"("error in (no error)"=w769, "VI ref"=w771, "refnum"=w772) -> ("error out"=w768:errorcluster, "refnum out"=w770:T17)  [unwired: 7 in]
                n441 = call <vilib>:"Close Config Data.vi"("error in (no error)"=w768, "refnum"=w770) -> ("error out"=w763:errorcluster, "file path"=w762:path)  [unwired: 8 in]
                n442 = Open/Create/Replace File(file path (use dialog)=w762, error in=w763) -> (refnum out=w766:refnum<file>, error out=w767:errorcluster)  [unwired: 4 in, 1 out]
                n443 = Flush File(refnum=w766, error in=w767) -> (refnum out=w765:refnum<file>, error out=w764:errorcluster)
                n444 = Close File(refnum=w765, error in=w764) -> ()  [unwired: 2 out]
              }
            }
          }
        }
      }
      event "仪器参数": Value Change {
        n445 = event-data() -> ()  [unwired: 1 in, 6 out]
        n446 = global read "总磷总氮断电保存全局变量.vi" "COD仪器参数"() -> (w778:T26)
        n447 = global read "总磷总氮断电保存全局变量.vi" "氨氮仪器参数"() -> (w777:T26)
        n448 = global read "总磷总氮断电保存全局变量.vi" "总氮仪器参数"() -> (w776:T26)
        n449 = global read "总磷总氮断电保存全局变量.vi" "总磷仪器参数"() -> (w775:T26)
        n450 = Bundle("COD仪器参数"=w778, "氨氮仪器参数"=w777, "总氮仪器参数"=w776, "总磷仪器参数"=w775) -> (w774:T27)  [unwired: 1 in]
        n451 = call "仪器参数设置.vi"("仪器参数"=w774) -> ("仪器参数 2"=w773:T27, "check？"=w779:bool)  [unwired: 9 in]
        n452 = case shown="真" w779 {
          tunnel: w773 -> [_ w780]
          frame False {
          }
          frame True {
            n453 = flat-sequence {
              tunnel: w780 -> [w785]
              frame #0 {
                n454 = Unbundle By Name(w785) -> ("COD仪器参数"=w783:T26, "氨氮仪器参数"=w782:T26, "总氮仪器参数"=w784:T26, "总磷仪器参数"=w781:T26)
                n455 = global write "总磷总氮断电保存全局变量.vi" "COD仪器参数"(w783) -> ()
                n456 = global write "总磷总氮断电保存全局变量.vi" "氨氮仪器参数"(w782) -> ()
                n457 = global write "总磷总氮断电保存全局变量.vi" "总氮仪器参数"(w784) -> ()
                n458 = global write "总磷总氮断电保存全局变量.vi" "总磷仪器参数"(w781) -> ()
              }
              frame #1 {
                n459 = call "配置文件路径.vi"() -> ("appended path"=w786:path)  [unwired: 11 in]
                n460 = call <vilib>:"Open Config Data.vi"("configuration file path"=w786) -> ("error out"=w794:errorcluster, "refnum"=w797:T17)  [unwired: 8 in, 1 out]
                n461 = vi-ref "总磷总氮断电保存全局变量.vi"() -> (w796:refnum<vi>)
                n462 = call <userlib>:"Write Panel to INI__ogtk.vi"("error in (no error)"=w794, "VI ref"=w796, "refnum"=w797) -> ("error out"=w793:errorcluster, "refnum out"=w795:T17)  [unwired: 7 in]
                n463 = call <vilib>:"Close Config Data.vi"("error in (no error)"=w793, "refnum"=w795) -> ("error out"=w788:errorcluster, "file path"=w787:path)  [unwired: 8 in]
                n464 = Open/Create/Replace File(file path (use dialog)=w787, error in=w788) -> (refnum out=w791:refnum<file>, error out=w792:errorcluster)  [unwired: 4 in, 1 out]
                n465 = Flush File(refnum=w791, error in=w792) -> (refnum out=w790:refnum<file>, error out=w789:errorcluster)
                n466 = Close File(refnum=w790, error in=w789) -> ()  [unwired: 2 out]
              }
            }
          }
        }
      }
      event "测试量程配置": Value Change {
        n467 = event-data() -> ()  [unwired: 1 in, 6 out]
        n468 = flat-sequence {
          tunnel: w798 -> [w801]
          frame #0 {
            n469 = property class="Enum (严格)"(reference=w801) -> ("Value"=w800:enum16{"COD", "氨氮", "总氮", "总磷"})  [unwired: 1 in, 2 out]
            n470 = case shown="默认" w800 {
              tunnel: "测试量程配置" -> [_ w802 w803 w804 w805]
              frame Default {
              }
              frame "COD" {
                n471 = global write "总磷总氮断电保存全局变量.vi" "COD自动测试量程配置"(w802) -> ()
              }
              frame "氨氮" {
                n472 = global write "总磷总氮断电保存全局变量.vi" "氨氮自动测试量程配置"(w803) -> ()
              }
              frame "总氮" {
                n473 = global write "总磷总氮断电保存全局变量.vi" "总氮自动测试量程配置"(w804) -> ()
              }
              frame "总磷" {
                n474 = global write "总磷总氮断电保存全局变量.vi" "总磷自动测试量程配置"(w805) -> ()
              }
            }
          }
          frame #1 {
            n475 = call "配置文件路径.vi"() -> ("appended path"=w806:path)  [unwired: 11 in]
            n476 = call <vilib>:"Open Config Data.vi"("configuration file path"=w806) -> ("error out"=w814:errorcluster, "refnum"=w817:T17)  [unwired: 8 in, 1 out]
            n477 = vi-ref "总磷总氮断电保存全局变量.vi"() -> (w816:refnum<vi>)
            n478 = call <userlib>:"Write Panel to INI__ogtk.vi"("error in (no error)"=w814, "VI ref"=w816, "refnum"=w817) -> ("error out"=w813:errorcluster, "refnum out"=w815:T17)  [unwired: 7 in]
            n479 = call <vilib>:"Close Config Data.vi"("error in (no error)"=w813, "refnum"=w815) -> ("error out"=w808:errorcluster, "file path"=w807:path)  [unwired: 8 in]
            n480 = Open/Create/Replace File(file path (use dialog)=w807, error in=w808) -> (refnum out=w811:refnum<file>, error out=w812:errorcluster)  [unwired: 4 in, 1 out]
            n481 = Flush File(refnum=w811, error in=w812) -> (refnum out=w810:refnum<file>, error out=w809:errorcluster)
            n482 = Close File(refnum=w810, error in=w809) -> ()  [unwired: 2 out]
          }
        }
      }
      event "手动启动": Value Change {
        n483 = event-data() -> ()  [unwired: 1 in, 6 out]
        n484 = call "总磷总氮启动参数对话框.vi"() -> ("确认"=w818:bool, "元素"=w819:cluster{"命令":string, "data":variant})  [unwired: 10 in]
        n485 = case shown="真" w818 {
          tunnel: w820 -> [_ w823]
          tunnel: w819 -> [_ w822]
          frame False {
          }
          frame True {
            n486 = Flush Queue(queue=w823) -> (queue out=w821:refnum<queue>)  [unwired: 1 in, 2 out]
            n487 = Enqueue Element(queue=w821, element=w822) -> ()  [unwired: 2 in, 3 out]
          }
        }
      }
      event "单步测试": Value Change {
        n488 = event-data() -> ()  [unwired: 1 in, 6 out]
        n489 = call "总磷单步调试对话框.vi"() -> ()  [unwired: 12 in]
      }
      event "停止": Value Change {
        n490 = event-data() -> ()  [unwired: 1 in, 6 out]
        n491 = Send Notification(notification=TRUE ("通知"), notifier=w825) -> ()  [unwired: 1 in, 2 out]
        n492 = Enqueue Element(queue=w829, element=cluster{"命令":string, "data":variant} {"命令"="启动", "data"=variant(cluster{"站号":u16, "控制命令输出":u16[]} {"站号"=1, "控制命令输出"=[2816]})} ("元素")) -> (queue out=w826:refnum<queue>)  [unwired: 2 in, 2 out]
        n493 = Enqueue Element(queue=w826, element=cluster{"命令":string, "data":variant} {"命令"="启动", "data"=variant(cluster{"站号":u16, "控制命令输出":u16[]} {"站号"=2, "控制命令输出"=[2816]})} ("元素")) -> ()  [unwired: 2 in, 3 out]
      }
      event "参数设置": Value Change {
        n494 = event-data() -> ()  [unwired: 1 in, 6 out]
        n495 = property on="窗格" class="Pane"("Origin"=T13 {"Horizontal"=0, "Vertical"=628} ("原点")) -> ()  [unwired: 2 in, 2 out]
      }
      event "返回": Value Change {
        n496 = event-data() -> ()  [unwired: 1 in, 6 out]
        n497 = property on="窗格" class="Pane"("Origin"=T13 {"Horizontal"=0, "Vertical"=0} ("原点")) -> ()  [unwired: 2 in, 2 out]
      }
      event "公式.X^2", "公式.X", "公式.b", "量程参数读取.测量精度", "量程参数读取.检出限", "量程参数读取.上限", "量程参数读取.下限", "量程参数读取.阈值（低->高）", "量程参数读取.阈值（高->低）", "量程参数读取.稀释度": Mouse Down {
        n498 = event-data() -> ("CtlRef"=w835:refnum<vi>)  [unwired: 1 in, 7 out]
        n499 = property class="DigNum (严格)"(reference=w835) -> (reference out=w833:refnum<vi>, "Value"=w834:dbl)  [unwired: 1 in, 1 out]
        n500 = call "数字键盘.vi"("OldNumber"=w834) -> ("NewNumber"=w832:dbl)
        n501 = property class="DigNum (严格)"(reference=w833, "Val(Sgnl)"=w832) -> ()  [unwired: 1 in, 2 out]
      }
      event "读公式": Value Change {
        n502 = event-data() -> ()  [unwired: 1 in, 6 out]
        n503 = property class="Enum (严格)"(reference=w843) -> ("Value"=w842:enum16{"COD", "氨氮", "总氮", "总磷"})  [unwired: 1 in, 2 out]
        n504 = property class="Enum (严格)"(reference=w844) -> ("Value"=w841:enum16{"水样测量", "零点核查", "跨度核查", "标样核查", "加标回收"})  [unwired: 1 in, 2 out]
        n505 = property class="Enum (严格)"(reference=w845) -> ("Value"=w840:enum16{"低量程", "高量程"})  [unwired: 1 in, 2 out]
        n506 = call "总磷总氮公式读取.vi"("量程"=w840, "测量模式"=w841, "测量参数"=w842) -> ("error out"=w837:errorcluster, "公式"=w838:cluster{"X^2":dbl, "X":dbl, "b":dbl})  [unwired: 7 in]
        n507 = property class="Clust (严格)"(reference=w839, "Value"=w838) -> ()  [unwired: 1 in, 2 out]
        n508 = case shown="错误" w837 {
          tunnel: ["读取成功" ("消息") "读取失败" ("消息")] -> w836
          frame No Error {
          }
          frame Error {
          }
        }
        n509 = One Button Dialog(message=w836) -> ()  [unwired: 1 in, 1 out]
      }
      event "写公式": Value Change {
        n510 = event-data() -> ()  [unwired: 1 in, 6 out]
        n511 = call "总磷总氮公式写入.vi"("公式"="公式", "量程"="量程下拉列表", "测量模式"="测量模式下拉列表", "测量参数"="参数下拉列表") -> ("error out"=w852:errorcluster)  [unwired: 7 in]
        n512 = case shown="无错误" w852 {
          tunnel: ["写入成功" ("消息") "写入失败" ("消息")] -> w853
          tunnel: "测量模式下拉列表" -> [w862 _]
          tunnel: "量程下拉列表" -> [w860 _]
          tunnel: "参数下拉列表" -> [w855 _]
          tunnel: "公式" -> [w854 _]
          frame No Error {
            n513 = Equal?(x=w862, y=enum16{"水样测量", "零点核查", "跨度核查", "标样核查", "加标回收"}."水样测量" ("测量模式下拉列表")) -> (x = y?=w858:bool)
            n514 = Equal?(x=w860, y=enum16{"低量程", "高量程"}."低量程" ("量程下拉列表")) -> (x = y?=w857:bool)
            n515 = And(x=w858, y=w857) -> (x .and. y?=w856:bool)
            n516 = case shown="真" w856 {
              tunnel: w855 -> [_ w865]
              tunnel: w854 -> [_ w864]
              frame False {
              }
              frame True {
                n517 = case shown="\"COD\"" w865 {
                  tunnel: w864 -> [w866 w872 w878 w884]
                  frame "总磷", Default {
                    n518 = Unbundle By Name(w866) -> ("X^2"=w869:dbl, "X"=w868:dbl, "b"=w867:dbl)
                    n519 = global read "总磷总氮断电保存全局变量.vi" "总磷仪器参数"() -> (w870:T26)
                    n520 = Bundle By Name(cluster=w870, "曲线截距"=w867, "曲线斜率"=w868, "二次多项式系数"=w869) -> (w871:T26)
                    n521 = global write "总磷总氮断电保存全局变量.vi" "总磷仪器参数"(w871) -> ()
                  }
                  frame "总氮" {
                    n522 = Unbundle By Name(w872) -> ("X^2"=w875:dbl, "X"=w874:dbl, "b"=w873:dbl)
                    n523 = global read "总磷总氮断电保存全局变量.vi" "总氮仪器参数"() -> (w876:T26)
                    n524 = Bundle By Name(cluster=w876, "曲线截距"=w873, "曲线斜率"=w874, "二次多项式系数"=w875) -> (w877:T26)
                    n525 = global write "总磷总氮断电保存全局变量.vi" "总氮仪器参数"(w877) -> ()
                  }
                  frame "COD" {
                    n526 = Unbundle By Name(w878) -> ("X^2"=w881:dbl, "X"=w880:dbl, "b"=w879:dbl)
                    n527 = global read "总磷总氮断电保存全局变量.vi" "COD仪器参数"() -> (w882:T26)
                    n528 = Bundle By Name(cluster=w882, "曲线截距"=w879, "曲线斜率"=w880, "二次多项式系数"=w881) -> (w883:T26)
                    n529 = global write "总磷总氮断电保存全局变量.vi" "COD仪器参数"(w883) -> ()
                  }
                  frame "氨氮" {
                    n530 = Unbundle By Name(w884) -> ("X^2"=w887:dbl, "X"=w886:dbl, "b"=w885:dbl)
                    n531 = global read "总磷总氮断电保存全局变量.vi" "氨氮仪器参数"() -> (w888:T26)
                    n532 = Bundle By Name(cluster=w888, "曲线截距"=w885, "曲线斜率"=w886, "二次多项式系数"=w887) -> (w889:T26)
                    n533 = global write "总磷总氮断电保存全局变量.vi" "氨氮仪器参数"(w889) -> ()
                  }
                }
              }
            }
          }
          frame Error {
          }
        }
        n534 = One Button Dialog(message=w853) -> ()  [unwired: 1 in, 1 out]
      }
      event "量程切换阈值读取": Value Change {
        n535 = event-data() -> ()  [unwired: 1 in, 6 out]
        n536 = property class="Enum (严格)"(reference=w896) -> ("Value"=w895:enum16{"COD", "氨氮", "总氮", "总磷"})  [unwired: 1 in, 2 out]
        n537 = call "总磷总氮量程读取.vi"("测量参数"=w895) -> ("error out"=w892:errorcluster, "量程参数读取"=w891:T28)  [unwired: 9 in]
        n538 = property class="Clust (严格)"(reference=w894, "Value"=w891) -> ()  [unwired: 1 in, 2 out]
        n539 = case shown="错误" w892 {
          tunnel: ["读取成功" ("消息") "读取失败" ("消息")] -> w893
          frame No Error {
          }
          frame Error {
          }
        }
        n540 = One Button Dialog(message=w893) -> ()  [unwired: 1 in, 1 out]
      }
      event "量程切换阈值写入": Value Change {
        n541 = event-data() -> ()  [unwired: 1 in, 6 out]
        n542 = property class="Enum (严格)"(reference=w903) -> ("Value"=w899:enum16{"COD", "氨氮", "总氮", "总磷"})  [unwired: 1 in, 2 out]
        n543 = call "总磷总氮量程写入.vi"("量程参数写入"="量程参数读取", "测量参数"=w899) -> ("error out"=w901:errorcluster)  [unwired: 8 in]
        n544 = case shown="无错误" w901 {
          tunnel: ["写入成功" ("消息") "写入失败" ("消息")] -> w902
          frame No Error {
          }
          frame Error {
          }
        }
        n545 = One Button Dialog(message=w902) -> ()  [unwired: 1 in, 1 out]
      }
    }
  }
